vi "rydberg_trigger_snap_2014_8_21_joe.vi"() -> ()   [LabVIEW 2013]
uses:
  AndorCamera/camera_controls.ctl
  <userlib>/atmcd32d.llb/AcquisitionMode_mode typedef.ctl
  <userlib>/atmcd32d.llb/TriggerMode_mode typedef.ctl
  instrumentvi_Neutral/cameratrigger/related_vi/check_pixelfly_status.vi
  <vilib>/Utility/file.llb/Write To Spreadsheet File (I64).vi
panel:
  in  "Num2Save":i32
  in  "Base Filename":string
  in  "Save Files?":bool
  out "appended path 2":path
  out "appended path":path
  in  "Case Constant\n(See Context Help) 2":bool
  in  "Case Constant\n(See Context Help)":bool
  out "iteration#":i32=25
  in  "Turn channels ON/OFF\n(works in real time)":bool[](array[boolean])=[TRUE, TRUE, FALSE, FALSE, FALSE, FALSE, FALSE, FALSE, FALSE, FALSE, FALSE, FALSE, FALSE, FALSE, FALSE, FALSE]
  in  "Save data every nth iteration":dbl=25.0
  out "Analog Input \nVoltage Monitor":T1(graph)={"data[0]"=-0.7588496337314492, "data[1]"=-0.07985869959699164, "data[2]"=0.0, "data[3]"=0.0, "data[4]"=0.0, "data[5]"=0.0, "data[6]"=0.0, "data[7]"=0.0, "data[8]"=0.0, "data[9]"=0.0, "data[10]"=0.0, "data[11]"=0.0, "data[12]"=0.0, "data[13]"=0.0, "data[14]"=0.0, "data[15]"=0.0}
  in  "Tab Control":enum32{"Controls", "Images", "Status"}(tab)=enum."Images"
  in  "Voltage Log File Path":path=path "C:/data/Voltage Log Files/voltagelog011708.txt"
  in  "Monitor voltages?":bool
  in  "Voltage\nMonitor\nControl":u16(ring)=1 caption="Voltage Monitor Control" items=["Off", "Each imaging cycle", "Verdi temp mon"]
  in  "File Path for Atoms":path=path "C:/data/tempfiles/junkatoms.dat"
  in  "File Path for Background":path=path "C:/data/tempfiles/junkback.dat"
  in  "Timeout (min 100 ms)":u32=1000
  in  "Max Iteration (timeout)":i32=51
  in  "Camera background with no image beam.\nIt will be subtracted before the log is taken":i16 min=0
  in  "Software Bin Size":i32=2
  in  "Software Binning?":bool=TRUE
  in  "Cut Image?":bool=TRUE
  in  "ROI Parameters":T2={"Col Start"=250, "Col Stop"=100, "Row Start"=1025, "Row stop"=1000} {"Row stop" min=1 max=1000; "Row Start" min=1 max=1000; "Col Stop" min=1 max=1000; "Col Start" min=1 max=1000}
  in  "Coil Current (amps)":dbl=34.0 format="%.2f"
  in  "Natural Linewidth of Transition (in MHz)":dbl=32.0
  in  "Image Beam Detuning (MHz)":dbl format="%.2f"
  in  "Image Beam Wavelength (m)":dbl=4.61e-07
  in  "Number for Scale":dbl=5.0
  in  "Number of Pixels to Smooth":dbl=1.0
  in  "Cut Borders":dbl
  in  "Limit":dbl=5.0
  in  "Sample Interleave":dbl=1.0 min=1.0
  in  "Pixel Size (m)":dbl=6e-06
  in  "Scale Base Level?":bool
  in  "1D Fit On?":bool=TRUE
  in  "2D Fit On?":bool=TRUE
  in  "Acquisition Parameters":T3={"Acquisition Mode"=enum."Kinetics", "Trigger Mode"=enum."External", "Frame \nTransfer"=FALSE, "Exposure Time (s)"=0.0001, "Accumulation Cycle Time (s)"=0.0, "# Accumulations"=1, "# Kinetics"=2, "Kinetic Cycle Time (s)"=0.0, "Horizontal Bin Size"=1, "Vertical Bin Size"=1} {"Vertical Bin Size" min=1; "Horizontal Bin Size" min=1; "Kinetic Cycle Time (s)" format="%.2f"; "# Kinetics" min=1; "# Accumulations" min=1; "Accumulation Cycle Time (s)" format="%.2f"; "Exposure Time (s)" format="%.2e"}
  out "Andor Initialize Error":errorcluster
  out "?":ext format="%.2f"
  in  "?":i32=35
  in  "?":i32=87
  out "PixelFly Status":bool
  out "Atoms - Background at Analysis Size":dbl[][](graph)
  out "image -  bg sum of ROI from back":dbl(graph)=-492168.0
  out "Last 40 numbers":dbl(graph)
  out "Atoms Image":i32[][](graph)
  out "Atoms - Background":i32[][](graph)
  out "parameters from \npeak absorption":T6={"alpha"=1.0152277070063695e-13, "peakdensity"=4.819850374584978e+17, "alphadenssigzsqrt2pi"=2.914507, "number"=142895.21998245403} {"number" format="%.3e"; "alphadenssigzsqrt2pi" format="%.3e"; "peakdensity" format="%.3e"; "alpha" format="%.3e"}
  out "Image Size for Analysis":i32[](array[numeric])=[150, 100]
  out "peak OD":dbl format="%#_4g"
  in  "# Images to Sum":i32=1
  in  "Continuous Scan?\n(No Images Saved)":bool=TRUE
  in  "Autoscale\nRoutine On?":bool
  in  "Analyze \nImages?":bool=TRUE
  in  "Camera Function":i32(ring)=2 items=["Camera Initialize", "Acquire", "Shutdown"]
  in  "Stop Continuous Scan?":bool
  out "2D Fit Chi-squared":dbl format="%#_3g"
  out "Num Atoms - OD Integral":dbl format="%#_4g"
  out "Num Atoms - Peak OD":dbl format="%#_4g"
  out "Y 1D Fit Values":T7={"Amplitude"=17.90491094333259, "y0"=0.0006453741239587313, "rmswidthy"=3.333942391455422e-05, "offsety"=-3.142553421752575, "Number Y"=176863.40216585185} {"Number Y" format="%.2e"; "offsety" format="%.2e"; "rmswidthy" format="%.2e"; "y0" format="%.2e"; "Amplitude" format="%.2e"}
  out "X 1D Fit Values":T8={"Amplitude"=24.47847782439825, "x0"=0.0009429207504454069, "rmswidthx"=2.376173376668835e-05, "offsetx"=-2.0737454877905925, "Number X"=172333.71575846447} {"Number X" format="%.2e"; "offsetx" format="%.2e"; "rmswidthx" format="%.2e"; "x0" format="%.2e"; "Amplitude" format="%.2e"}
  out "2-D Fit Parameters":T9
  out "Avg Back":ext=1449.7175567626953 format="%.2e"
  out "Avg Atoms-Back":ext=-7.78399887084961 format="%.2e"
  out "Avg Atoms":ext=1441.9335578918458 format="%.2e"
  out "Opticaldepthimagesingle (ln(atoms)-ln(back))(-1)":dbl[][](graph)
  out "Smoothed OD - Fit OD":dbl[][](graph)
  out "Uncut Image - Doubleshot":i32[][](graph)
  out "Y density distribution: log(sum_x atoms) -log(sum_x backgnd)":cluster{dbl[], dbl[]}[](graph)=[{[0.0, 1.2e-05, 2.4e-05, 3.6e-05, 4.8e-05, 6e-05, 7.2e-05, 8.400000000000001e-05, 9.6e-05, 0.000108, 0.00012, 0.000132, 0.000144, 0.000156, 0.00016800000000000002, 0.00018, 0.000192, 0.000204, 0.000216, 0.000228, 0.00024, 0.000252, 0.000264, 0.000276, 0.000288, 0.00030000000000000003, 0.000312, 0.000324, 0.00033600000000000004, 0.000348, 0.00036, 0.000372, 0.000384, 0.00039600000000000003, 0.000408, 0.00042, 0.000432, 0.000444, 0.000456, 0.000468, 0.00048, 0.000492, 0.000504, 0.000516, 0.000528, 0.00054, 0.000552, 0.000564, 0.000576, 0.000588, 0.0006000000000000001, 0.000612, 0.000624, 0.0006360000000000001, 0.000648, 0.00066, 0.0006720000000000001, 0.000684, 0.000696, 0.000708, 0.00072, 0.000732, 0.000744, 0.000756, 0.000768, 0.00078, 0.0007920000000000001, 0.000804, 0.000816, 0.0008280000000000001, 0.00084, 0.000852, 0.000864, 0.000876, 0.000888, 0.0009, 0.000912, 0.000924, 0.000936, 0.0009480000000000001, 0.00096, 0.000972, 0.000984, 0.000996, 0.001008, 0.00102, 0.001032, 0.001044, 0.001056, 0.001068, 0.00108, 0.001092, 0.001104, 0.001116, 0.001128, 0.00114, 0.001152, 0.001164, 0.001176, 0.001188], [-3.3686591448665695, -3.3593416907117444, -2.501141797799619, -3.137266718233832, -3.587719306130566, -2.6390745848241295, -3.6966092446853054, -2.6808187998242374, -3.0319112156403207, -2.7363781603955886, -3.363138854673707, -2.731002614818408, -3.3935197594450983, -3.0493035465378853, -3.2941032756557433, -3.092209549305835, -3.0943983454935733, -3.2393686037710268, -2.730035543135955, -3.287849371356515, -2.5686023814239434, -3.1088703551167782, -2.856653458062283, -3.240447915604136, -3.4894394818825276, -2.9961131164766357, -4.104169957056229, -2.8255474959485127, -3.8878748767015168, -3.0775415698653887, -3.7197529539632797, -3.3776657935209187, -3.8047169273982036, -3.4536401406066943, -3.3930728929356064, -3.1293918380520154, -3.433923718918095, -2.8153587940721536, -3.6029531308467995, -2.4989306176071295, -3.483829652183431, -2.9711985693618317, -3.697510544320039, -3.1132099718149675, -3.803881645787669, -3.6495652439025434, -3.6485837854809233, -3.185441611433589, -1.652208255575033, 0.03140941165247568, 4.4569342541294645, 8.56173788023807, 12.377374823114451, 13.49419715605518, 13.361094012986996, 13.08877719779457, 10.635138116352437, 6.592571400876977, 2.8347368854219894, -0.6335944505865427, -2.5137500326873123, -3.043489857024497, -2.68801842384687, -3.0676047259767074, -2.9163649829733913, -3.168337622954141, -2.7690334242099652, -3.322776293644665, -3.119521162448791, -3.04783132514558, -2.619550840819329, -3.2013707187938962, -2.419650797146687, -2.902692626093767, -3.0917951318126597, -2.8856469922691304, -3.523759843666312, -3.0084041621928463, -3.646833134218241, -3.1529925921761333, -3.371597483779624, -3.5211395371050003, -3.153552371623391, -3.4981555573237983, -3.7751962171532796, -2.992402620435996, -3.2399196976318763, -2.831696410884433, -2.7750651929482046, -2.8873123361618127, -2.360377205045097, -2.399998629312904, -2.590436576132106, -2.2120804438281993, -2.5532249988086733, -2.7154620505466482, -2.369902307173561, -3.201516908291751, -2.571788439326383, -2.629373703639885]}, {[0.0, 1.2e-05, 2.4e-05, 3.6e-05, 4.8e-05, 6e-05, 7.2e-05, 8.400000000000001e-05, 9.6e-05, 0.000108, 0.00012, 0.000132, 0.000144, 0.000156, 0.00016800000000000002, 0.00018, 0.000192, 0.000204, 0.000216, 0.000228, 0.00024, 0.000252, 0.000264, 0.000276, 0.000288, 0.00030000000000000003, 0.000312, 0.000324, 0.00033600000000000004, 0.000348, 0.00036, 0.000372, 0.000384, 0.00039600000000000003, 0.000408, 0.00042, 0.000432, 0.000444, 0.000456, 0.000468, 0.00048, 0.000492, 0.000504, 0.000516, 0.000528, 0.00054, 0.000552, 0.000564, 0.000576, 0.000588, 0.0006000000000000001, 0.000612, 0.000624, 0.0006360000000000001, 0.000648, 0.00066, 0.0006720000000000001, 0.000684, 0.000696, 0.000708, 0.00072, 0.000732, 0.000744, 0.000756, 0.000768, 0.00078, 0.0007920000000000001, 0.000804, 0.000816, 0.0008280000000000001, 0.00084, 0.000852, 0.000864, 0.000876, 0.000888, 0.0009, 0.000912, 0.000924, 0.000936, 0.0009480000000000001, 0.00096, 0.000972, 0.000984, 0.000996, 0.001008, 0.00102, 0.001032, 0.001044, 0.001056, 0.001068, 0.00108, 0.001092, 0.001104, 0.001116, 0.001128, 0.00114, 0.001152, 0.001164, 0.001176, 0.001188], [-3.142553421752575, -3.142553421752575, -3.142553421752575, -3.142553421752575, -3.142553421752575, -3.142553421752575, -3.142553421752575, -3.142553421752575, -3.142553421752575, -3.142553421752575, -3.142553421752575, -3.142553421752575, -3.142553421752575, -3.142553421752575, -3.142553421752575, -3.142553421752575, -3.142553421752575, -3.142553421752575, -3.142553421752575, -3.142553421752575, -3.142553421752575, -3.142553421752575, -3.142553421752575, -3.142553421752575, -3.142553421752575, -3.142553421752575, -3.142553421752575, -3.142553421752575, -3.142553421752575, -3.142553421752575, -3.142553421752573, -3.14255342175253, -3.1425534217517685, -3.1425534217398705, -3.1425534215767574, -3.142553419615115, -3.142553398924452, -3.142553207572838, -3.1425516564361646, -3.1425406396371858, -3.1424721164431455, -3.1420990921048606, -3.1403231424865408, -3.1329354518498045, -3.106116340729864, -3.021287229549591, -2.788007984145684, -2.231927393950265, -1.0878733189191243, 0.9301648516208109, 3.9493125759985808, 7.706020947338827, 11.43621434642004, 14.068401345797076, 14.706907582526853, 13.11971957540532, 9.873322089660576, 6.009141262246697, 2.510273096557114, -0.0751860764137236, -1.680369782741332, -2.530239620690055, -2.917294410160682, -3.0697542735255157, -3.1218850426129303, -3.137398494519852, -3.1414239518658547, -3.1423360201347044, -3.1425166607891493, -3.1425479610692, -3.1425527091570276, -3.142553340061387, -3.1425534135255404, -3.142553421024716, -3.1425534216960047, -3.1425534217487128, -3.142553421752343, -3.142553421752563, -3.1425534217525746, -3.142553421752575, -3.142553421752575, -3.142553421752575, -3.142553421752575, -3.142553421752575, -3.142553421752575, -3.142553421752575, -3.142553421752575, -3.142553421752575, -3.142553421752575, -3.142553421752575, -3.142553421752575, -3.142553421752575, -3.142553421752575, -3.142553421752575, -3.142553421752575, -3.142553421752575, -3.142553421752575, -3.142553421752575, -3.142553421752575, -3.142553421752575]}]
  out "Intensity v/s X":cluster{dbl[], dbl[]}[](graph)=[{[0.0, 1.2e-05, 2.4e-05, 3.6e-05, 4.8e-05, 6e-05, 7.2e-05, 8.400000000000001e-05, 9.6e-05, 0.000108, 0.00012, 0.000132, 0.000144, 0.000156, 0.00016800000000000002, 0.00018, 0.000192, 0.000204, 0.000216, 0.000228, 0.00024, 0.000252, 0.000264, 0.000276, 0.000288, 0.00030000000000000003, 0.000312, 0.000324, 0.00033600000000000004, 0.000348, 0.00036, 0.000372, 0.000384, 0.00039600000000000003, 0.000408, 0.00042, 0.000432, 0.000444, 0.000456, 0.000468, 0.00048, 0.000492, 0.000504, 0.000516, 0.000528, 0.00054, 0.000552, 0.000564, 0.000576, 0.000588, 0.0006000000000000001, 0.000612, 0.000624, 0.0006360000000000001, 0.000648, 0.00066, 0.0006720000000000001, 0.000684, 0.000696, 0.000708, 0.00072, 0.000732, 0.000744, 0.000756, 0.000768, 0.00078, 0.0007920000000000001, 0.000804, 0.000816, 0.0008280000000000001, 0.00084, 0.000852, 0.000864, 0.000876, 0.000888, 0.0009, 0.000912, 0.000924, 0.000936, 0.0009480000000000001, 0.00096, 0.000972, 0.000984, 0.000996, 0.001008, 0.00102, 0.001032, 0.001044, 0.001056, 0.001068, 0.00108, 0.001092, 0.001104, 0.001116, 0.001128, 0.00114, 0.001152, 0.001164, 0.001176, 0.001188, 0.0012000000000000001, 0.001212, 0.001224, 0.0012360000000000001, 0.001248, 0.00126, 0.0012720000000000001, 0.001284, 0.001296, 0.0013080000000000001, 0.00132, 0.001332, 0.0013440000000000001, 0.001356, 0.001368, 0.00138, 0.001392, 0.001404, 0.001416, 0.001428, 0.00144, 0.001452, 0.001464, 0.001476, 0.001488, 0.0015, 0.001512, 0.001524, 0.001536, 0.0015480000000000001, 0.00156, 0.001572, 0.0015840000000000001, 0.001596, 0.001608, 0.0016200000000000001, 0.001632, 0.001644, 0.0016560000000000001, 0.001668, 0.00168, 0.0016920000000000001, 0.001704, 0.001716, 0.001728, 0.00174, 0.001752, 0.001764, 0.001776, 0.001788], [-2.8183440721355737, -2.401522563761773, -2.5237601060707675, -2.500570399573121, -2.506086929574394, -2.3798757992705077, -2.491986345524083, -2.488259685244998, -2.5954764602082605, -2.6088044268195745, -2.565883062250009, -2.640123527845276, -2.5258645679890606, -2.542319425147525, -2.3663141562295777, -2.491158449081013, -2.4827761290987382, -2.5697565230360624, -2.675555471134544, -2.4526500510070264, -2.587401679302161, -2.7170704998887913, -2.5610989943488676, -2.5911334487145723, -2.5002374964478804, -2.4884694389456854, -2.5394904176372393, -2.5500867554972046, -2.378216817131488, -2.5395407567208395, -2.046418844121149, -2.1733857420010736, -2.669858427788313, -2.2304504062857404, -2.586975439308276, -2.4213636413369386, -2.3929041134997533, -2.488418399790703, -2.2930625821045396, -2.6069475160815045, -2.511643300766991, -2.273400532704045, -2.2899489155247466, -2.528198542008795, -2.357612131615724, -2.3432177912642373, -2.3168511287027513, -2.420032372065748, -2.395414080287992, -2.3757390661600084, -2.4716707833126748, -2.2185297028257764, -2.2814791274250865, -2.118623996360043, -2.0182357551965424, -2.432618062946176, -2.230506420081042, -2.146155705062938, -2.3472190640306962, -2.3712543536693147, -2.1875881775472408, -2.1952908358917966, -2.053287952368919, -1.8502300747721847, -1.9848473505809352, -1.9942680470508094, -2.0174521250165753, -2.0969782433525097, -1.8219170436304921, -1.6672326334789886, -1.4869217102946095, -0.9996339197143698, -0.8098748137616667, -0.35967428953222225, -0.650012388682967, 1.7919178156766975, 7.743635801250548, 16.428591835436464, 22.663725551287143, 20.240706904645776, 16.936256193013378, 9.701135845766885, 4.174916332451744, -0.2899352730639748, -1.661331740025389, -1.5080821335172914, -1.9026215949503467, -2.049002401491748, -1.9706402437938095, -2.0311585837459916, -2.077597516112178, -1.930667645093763, -2.1086022731634557, -1.7650030212055299, -1.917311464733416, -1.8111299981898128, -2.075459160990931, -2.2079166808241553, -1.8235763980834463, -1.898222513860219, -1.9621602868612626, -2.0017564868267073, -1.7095965014406147, -2.0323342222595784, -1.6211606697328307, -1.839833902685882, -1.9658503587635323, -1.9776012347161895, -1.887885369120113, -1.9468724100556756, -1.6351243930344026, -1.6613815392586275, -1.6219275265368651, -1.7589024364108354, -1.6045421848466503, -1.8391976965150434, -1.6203149700231734, -1.7969550536250836, -1.5575704192364128, -1.8258635266791998, -1.9097093493073771, -1.8343058761104203, -1.660627277068329, -1.945166122309729, -1.5463727138680952, -1.569489672727741, -1.6225878206881816, -1.7324496472705277, -1.631544148883222, -1.8227215123275755, -1.8797703918872912, -1.8647363562896544, -1.576905869043685, -1.970412155507347, -2.0096411488008243, -1.7813961287674829, -1.8489792019571496, -1.7513334844093151, -1.6826445124467, -1.8905109948545942, -1.7110939804845202, -1.7394070082149256, -1.599355827269278, -1.686777376633131, -1.4884369858077662, -1.653664890583741, -1.8092625318996625, -1.4833808568982931, -1.6619157448002397, -1.371210367738854]}, {[0.0, 1.2e-05, 2.4e-05, 3.6e-05, 4.8e-05, 6e-05, 7.2e-05, 8.400000000000001e-05, 9.6e-05, 0.000108, 0.00012, 0.000132, 0.000144, 0.000156, 0.00016800000000000002, 0.00018, 0.000192, 0.000204, 0.000216, 0.000228, 0.00024, 0.000252, 0.000264, 0.000276, 0.000288, 0.00030000000000000003, 0.000312, 0.000324, 0.00033600000000000004, 0.000348, 0.00036, 0.000372, 0.000384, 0.00039600000000000003, 0.000408, 0.00042, 0.000432, 0.000444, 0.000456, 0.000468, 0.00048, 0.000492, 0.000504, 0.000516, 0.000528, 0.00054, 0.000552, 0.000564, 0.000576, 0.000588, 0.0006000000000000001, 0.000612, 0.000624, 0.0006360000000000001, 0.000648, 0.00066, 0.0006720000000000001, 0.000684, 0.000696, 0.000708, 0.00072, 0.000732, 0.000744, 0.000756, 0.000768, 0.00078, 0.0007920000000000001, 0.000804, 0.000816, 0.0008280000000000001, 0.00084, 0.000852, 0.000864, 0.000876, 0.000888, 0.0009, 0.000912, 0.000924, 0.000936, 0.0009480000000000001, 0.00096, 0.000972, 0.000984, 0.000996, 0.001008, 0.00102, 0.001032, 0.001044, 0.001056, 0.001068, 0.00108, 0.001092, 0.001104, 0.001116, 0.001128, 0.00114, 0.001152, 0.001164, 0.001176, 0.001188, 0.0012000000000000001, 0.001212, 0.001224, 0.0012360000000000001, 0.001248, 0.00126, 0.0012720000000000001, 0.001284, 0.001296, 0.0013080000000000001, 0.00132, 0.001332, 0.0013440000000000001, 0.001356, 0.001368, 0.00138, 0.001392, 0.001404, 0.001416, 0.001428, 0.00144, 0.001452, 0.001464, 0.001476, 0.001488, 0.0015, 0.001512, 0.001524, 0.001536, 0.0015480000000000001, 0.00156, 0.001572, 0.0015840000000000001, 0.001596, 0.001608, 0.0016200000000000001, 0.001632, 0.001644, 0.0016560000000000001, 0.001668, 0.00168, 0.0016920000000000001, 0.001704, 0.001716, 0.001728, 0.00174, 0.001752, 0.001764, 0.001776, 0.001788], [-2.0737454877905925, -2.0737454877905925, -2.0737454877905925, -2.0737454877905925, -2.0737454877905925, -2.0737454877905925, -2.0737454877905925, -2.0737454877905925, -2.0737454877905925, -2.0737454877905925, -2.0737454877905925, -2.0737454877905925, -2.0737454877905925, -2.0737454877905925, -2.0737454877905925, -2.0737454877905925, -2.0737454877905925, -2.0737454877905925, -2.0737454877905925, -2.0737454877905925, -2.0737454877905925, -2.0737454877905925, -2.0737454877905925, -2.0737454877905925, -2.0737454877905925, -2.0737454877905925, -2.0737454877905925, -2.0737454877905925, -2.0737454877905925, -2.0737454877905925, -2.0737454877905925, -2.0737454877905925, -2.0737454877905925, -2.0737454877905925, -2.0737454877905925, -2.0737454877905925, -2.0737454877905925, -2.0737454877905925, -2.0737454877905925, -2.0737454877905925, -2.0737454877905925, -2.0737454877905925, -2.0737454877905925, -2.0737454877905925, -2.0737454877905925, -2.0737454877905925, -2.0737454877905925, -2.0737454877905925, -2.0737454877905925, -2.0737454877905925, -2.0737454877905925, -2.0737454877905925, -2.0737454877905925, -2.0737454877905925, -2.0737454877905925, -2.0737454877905925, -2.0737454877905925, -2.0737454877905925, -2.0737454877905925, -2.0737454877905925, -2.0737454877905925, -2.0737454877905925, -2.073745487790578, -2.073745487789698, -2.073745487748773, -2.0737454862751323, -2.073745445235809, -2.0737445618346193, -2.073729875366191, -2.073541507399717, -2.0716803713160936, -2.0575446026371003, -1.9752602822028478, -1.6098273966897678, -0.3803839855887031, 2.715820000636734, 8.423627049166667, 15.754276644617699, 21.388186935825832, 21.85183342897553, 16.8322343699678, 9.50266684232387, 3.41896670995723, -0.05427383695049559, -1.4984026137046382, -1.9467308492977926, -2.052017531704562, -2.0708652918518737, -2.0734496434587752, -2.0737219404138356, -2.0737440354787706, -2.073745418381675, -2.073745485220145, -2.0737454877168293, -2.073745487788952, -2.073745487790564, -2.073745487790592, -2.0737454877905925, -2.0737454877905925, -2.0737454877905925, -2.0737454877905925, -2.0737454877905925, -2.0737454877905925, -2.0737454877905925, -2.0737454877905925, -2.0737454877905925, -2.0737454877905925, -2.0737454877905925, -2.0737454877905925, -2.0737454877905925, -2.0737454877905925, -2.0737454877905925, -2.0737454877905925, -2.0737454877905925, -2.0737454877905925, -2.0737454877905925, -2.0737454877905925, -2.0737454877905925, -2.0737454877905925, -2.0737454877905925, -2.0737454877905925, -2.0737454877905925, -2.0737454877905925, -2.0737454877905925, -2.0737454877905925, -2.0737454877905925, -2.0737454877905925, -2.0737454877905925, -2.0737454877905925, -2.0737454877905925, -2.0737454877905925, -2.0737454877905925, -2.0737454877905925, -2.0737454877905925, -2.0737454877905925, -2.0737454877905925, -2.0737454877905925, -2.0737454877905925, -2.0737454877905925, -2.0737454877905925, -2.0737454877905925, -2.0737454877905925, -2.0737454877905925, -2.0737454877905925, -2.0737454877905925, -2.0737454877905925, -2.0737454877905925, -2.0737454877905925, -2.0737454877905925, -2.0737454877905925]}] caption="X Density Distribution: log(sum_y atoms) -log(sum_y backgnd)"
  out "Background Image":i32[][](graph)
  out "Strip Chart\nerror out":errorcluster
  in  "Strip Chart\nerror in":errorcluster
  out "Strip chart counter":dbl
  out "error out":errorcluster={"status"=TRUE, "code"=-131, "source"="Remove buffer from list.vi: Picture buffer already in use"} caption="Camera Error Out 1"
  out "V bin 2":i32(ring) items=["1", "2"]
  out "H bin 2":i32(ring) items=["1", "2"]
  out "Size":i32=5242880
  out "Camera Information":T10 {"VS Speed (us)" format="%.2f"}
  out "Output ClusterY\n(arb fit)":T11={"amplitudey"=0.008995711509471623, "temperaturey"=0.002709094402736608, "alphay"=0.0011778671316246122, "offsety"=-0.0002344292151486787, "numbery"=771798750.645837, "peakdensityy"=4696134676573208.0, "centery"=0.004923587672892697} {"centery" format="%.2e"; "peakdensityy" format="%.2e"; "numbery" format="%.2e"; "offsety" format="%.2e"; "alphay" format="%.2e"; "temperaturey" format="%.2e"; "amplitudey" format="%.2e"}
  out "Output Cluster X\n(arb fit)":T12={"amplitudex"=0.0047697219685124154, "temperaturex"=0.0023439442598952344, "alphax"=0.0010191061999544498, "offsetx"=8.440276213188199e-05, "numberx"=708132868.1536969, "peakdensityx"=6652452808873044.0, "centerx"=0.0037182148271134325} {"centerx" format="%.2e"; "peakdensityx" format="%.2e"; "numberx" format="%.2e"; "offsetx" format="%.2e"; "alphax" format="%.2e"; "temperaturex" format="%.2e"; "amplitudex" format="%.2e"}
  out "Y side(by arbfit)":cluster{cluster{dbl, dbl}[]}[](graph)=[{[{0.0, -9.666143798828125e-05}, {4.63e-05, 4.321251220703125e-05}, {9.26e-05, -0.00016961046142578126}, {0.00013890000000000002, -0.0001606823974609375}, {0.0001852, -3.920782470703125e-05}, {0.0002315, -0.000111915087890625}, {0.00027780000000000003, -0.00018772257080078126}, {0.0003241, -0.00014607723388671877}, {0.0003704, 3.730218505859375e-05}, {0.0004167, -0.000120493310546875}, {0.000463, -2.0831201171875e-05}, {0.0005093, 8.1265576171875e-05}, {0.0005556000000000001, -4.6981127929687503e-05}, {0.0006019, 2.730753173828125e-05}, {0.0006482, 0.0001042299560546875}, {0.0006945, 8.897061767578125e-05}, {0.0007408, -0.0001128991943359375}, {0.0007871, -3.39658935546875e-05}, {0.0008334, 0.00021708648681640627}, {0.0008797, 1.521951904296875e-05}, {0.000926, -8.81429443359375e-05}, {0.0009723, 0.00017849017333984376}, {0.0010186, 0.00016118013916015624}, {0.0010649, 4.3130029296875e-05}, {0.0011112000000000001, 0.000101584814453125}, {0.0011575000000000001, 0.0001667121826171875}, {0.0012038, 0.0001330364013671875}, {0.0012501, 1.435771484375e-05}, {0.0012964, 0.00013017509765625}, {0.0013427, 0.0001979874267578125}, {0.001389, 0.0001995517578125}, {0.0014353, 5.386134033203125e-05}, {0.0014816, 0.00013825557861328125}, {0.0015279, 0.00037487060546875003}, {0.0015742, 0.0001915253173828125}, {0.0016205, 0.000173282373046875}, {0.0016668, 0.00030387272949218753}, {0.0017131, 0.0005522344604492188}, {0.0017594, 0.0003743757080078125}, {0.0018057, 0.000244183544921875}, {0.001852, 0.0004390764404296875}, {0.0018983000000000001, 0.0004536360961914063}, {0.0019446, 0.00044938680419921874}, {0.0019909, 0.00031516435546875}, {0.0020372, 0.0003973002685546875}, {0.0020835, 0.000558414990234375}, {0.0021298, 0.0005315966674804687}, {0.0021761, 0.00047105989990234374}, {0.0022224000000000002, 0.0006024039794921875}, {0.0022687000000000002, 0.0006190456176757812}, {0.0023150000000000002, 0.0006605089233398438}, {0.0023613, 0.0006151063476562501}, {0.0024076, 0.0007049785888671875}, {0.0024539, 0.0008554387939453125}, {0.0025002, 0.000755099755859375}, {0.0025465, 0.0008008635498046875}, {0.0025928, 0.0007846542358398437}, {0.0026391, 0.00092633427734375}, {0.0026854, 0.0009349409423828125}, {0.0027317, 0.0009390679321289063}, {0.002778, 0.0009715178466796875}, {0.0028243, 0.0009944736938476563}, {0.0028706, 0.001180484033203125}, {0.0029169, 0.0010933195068359375}, {0.0029632, 0.0010906231689453126}, {0.0030095, 0.0010906317016601563}, {0.0030558, 0.0013240981567382813}, {0.0031021, 0.0014536930297851564}, {0.0031484, 0.001447785546875}, {0.0031947, 0.0013987793212890626}, {0.003241, 0.0015179443725585938}, {0.0032873, 0.0015591374755859375}, {0.0033336, 0.0016731800537109376}, {0.0033799, 0.0016079417602539064}, {0.0034262, 0.0015991075561523438}, {0.0034725, 0.0018513971801757813}, {0.0035188, 0.0018405805419921875}, {0.0035651, 0.0018605926025390626}, {0.0036114, 0.001904240283203125}, {0.0036577, 0.0018782012817382813}, {0.003704, 0.0019519751342773437}, {0.0037503000000000002, 0.0020929782470703127}, {0.0037966000000000002, 0.002198195153808594}, {0.0038429000000000002, 0.0021514216552734377}, {0.0038892, 0.0020961069091796876}, {0.0039355, 0.002265489831542969}, {0.0039818, 0.0023468663330078127}, {0.0040281, 0.002427193310546875}, {0.0040744, 0.0024689637939453125}, {0.0041207, 0.0024438804565429686}, {0.004167, 0.0024601580322265626}, {0.0042133, 0.002636688525390625}, {0.0042596, 0.002699147998046875}, {0.0043059, 0.002643045397949219}, {0.0043522, 0.0026505143676757814}, {0.0043985, 0.0026222966796875}, {0.0044448000000000005, 0.0027097114990234377}, {0.0044911000000000005, 0.0027219531005859376}, {0.0045374000000000005, 0.0027993960205078125}, {0.0045837000000000004, 0.002850597998046875}, {0.0046300000000000004, 0.0028023995361328127}, {0.0046763, 0.0027945295288085937}, {0.0047226, 0.0029437581787109374}, {0.0047689, 0.0029110010864257813}, {0.0048152, 0.0030008591064453125}, {0.0048615, 0.002974151708984375}, {0.0049078, 0.002937995751953125}, {0.0049541, 0.0029096813598632814}, {0.0050004, 0.0029673767333984378}, {0.0050467, 0.003066478527832031}, {0.005093, 0.00306333564453125}, {0.0051393, 0.003041998168945313}, {0.0051856, 0.0028867596435546874}, {0.0052319, 0.0027757006713867187}, {0.0052782, 0.0028882158935546877}, {0.0053245, 0.0029104151733398437}, {0.0053708, 0.0027892534667968752}, {0.0054171, 0.0027464476806640624}, {0.0054634, 0.002764500061035156}, {0.0055097, 0.0026023215942382813}, {0.005556, 0.0025186128173828124}, {0.0056023, 0.002569339807128906}, {0.0056486, 0.0024484426147460938}, {0.0056949, 0.0024748428344726564}, {0.0057412, 0.002454739758300781}, {0.0057875, 0.0023008465576171877}, {0.0058338, 0.0023179062988281252}, {0.0058801, 0.00228233056640625}, {0.0059264, 0.0022157355712890624}, {0.0059727, 0.0020830091918945313}, {0.006019, 0.002083563818359375}, {0.0060653, 0.0020847953735351563}, {0.0061116, 0.002062195056152344}, {0.0061579, 0.0019736823608398437}, {0.0062042, 0.0018520598876953125}, {0.0062505, 0.0018948542968750001}, {0.0062968, 0.0017422921997070314}, {0.0063431, 0.0016028676391601562}, {0.0063894, 0.0016803645996093751}, {0.0064357, 0.0015904127197265625}, {0.006482, 0.0015004665283203126}, {0.0065283, 0.001450151953125}, {0.0065746, 0.0014172981567382812}, {0.0066209, 0.001336484814453125}, {0.0066672, 0.00135934111328125}, {0.0067135, 0.001208789892578125}, {0.0067598, 0.0012902744750976562}, {0.0068061, 0.0011487451782226563}, {0.0068524, 0.001103211767578125}, {0.0068987, 0.0011628611328125}, {0.006945, 0.0011180217163085937}, {0.0069913, 0.00104233369140625}, {0.0070376, 0.001006120849609375}, {0.0070839, 0.0009368323608398438}, {0.0071302, 0.0008879626586914063}, {0.0071765, 0.0008855393676757813}, {0.0072228, 0.0007939548950195313}, {0.0072691, 0.0007488623413085938}, {0.0073154, 0.0007369250732421875}, {0.0073617, 0.0007228916015625}, {0.007408, 0.0006716412719726563}, {0.0074543000000000005, 0.0006353601684570313}, {0.0075006000000000005, 0.0006309515991210938}, {0.0075469000000000005, 0.0005209734375}, {0.0075932000000000005, 0.0005503174438476563}, {0.0076395000000000005, 0.0005640096069335937}, {0.0076858000000000004, 0.0005803668212890625}, {0.0077321, 0.00046943583984375}, {0.0077784, 0.0004919138549804688}, {0.0078247, 0.0004567334716796875}, {0.007871, 0.0004032162841796875}, {0.0079173, 0.0003256823486328125}, {0.0079636, 0.00034895675048828126}, {0.0080099, 0.0002296722412109375}, {0.0080562, 0.00032278122558593753}, {0.0081025, 0.00024264196777343752}, {0.0081488, 0.0002704131103515625}, {0.0081951, 0.0002514306640625}, {0.0082414, 0.00023038614501953125}, {0.0082877, 0.00023180257568359376}]}, {[{0.0, -0.00010865906187833456}, {4.63e-05, -0.00010248175881259633}, {9.26e-05, -9.60946713894237e-05}, {0.00013890000000000002, -8.949093944564066e-05}, {0.0001852, -8.266349606890666e-05}, {0.0002315, -7.560506264006202e-05}, {0.00027780000000000003, -6.830814386093194e-05}, {0.0003241, -6.076502277862111e-05}, {0.0003704, -5.296775581859711e-05}, {0.0004167, -4.4908167840241404e-05}, {0.000463, -3.657784723005229e-05}, {0.0005093, -2.7968141049325046e-05}, {0.0005556000000000001, -1.9070150254923014e-05}, {0.0006019, -9.874725013701312e-06}, {0.0006482, -3.724601332668094e-07}, {0.0006945, 9.446309365930862e-06}, {0.0007408, 1.9591512509667256e-05}, {0.0007871, 3.0073346429921213e-05}, {0.0008334, 4.090228019253389e-05}, {0.0008797, 5.2089058356076504e-05}, {0.000926, 6.364470422192584e-05}, {0.0009723, 7.558052273170855e-05}, {0.0010186, 8.79081029641e-05}, {0.0010649, 0.00010063932017842472}, {0.0011112000000000001, 0.00011378633734756733}, {0.0011575000000000001, 0.0001273616061173385}, {0.0012038, 0.00014137786712360722}, {0.0012501, 0.00015584814959217083}, {0.0012964, 0.00017078577013944924}, {0.0013427, 0.0001862043306846068}, {0.001389, 0.00020211771537558232}, {0.0014353, 0.00021854008642268471}, {0.0014816, 0.00023548587872383942}, {0.0015279, 0.00025296979315517985}, {0.0015742, 0.00027100678838941274}, {0.0016205, 0.00028961207109216836}, {0.0016668, 0.00030880108433330974}, {0.0017131, 0.00032858949403583845}, {0.0017594, 0.0003489931732695157}, {0.0018057, 0.00037002818417953464}, {0.001852, 0.0003917107573224413}, {0.0018983000000000001, 0.00041405726816191505}, {0.0019446, 0.00043708421045589795}, {0.0019909, 0.00046080816624380496}, {0.0020372, 0.00048524577211806353}, {0.0020835, 0.0005104136814379354}, {0.0021298, 0.0005363285221153792}, {0.0021761, 0.0005630068495725409}, {0.0022224000000000002, 0.0005904650944382619}, {0.0022687000000000002, 0.0006187195045167119}, {0.0023150000000000002, 0.0006477860805248956}, {0.0023613, 0.0006776805050573274}, {0.0024076, 0.0007084180641957342}, {0.0024539, 0.000740013561139293}, {0.0025002, 0.0007724812211868801}, {0.0025465, 0.0008058345873573525}, {0.0025928, 0.0008400864058874109}, {0.0026391, 0.0008752485007996484}, {0.0026854, 0.0009113316366866587}, {0.0027317, 0.0009483453688115168}, {0.002778, 0.0009862978795816956}, {0.0028243, 0.0010251958004140647}, {0.0028706, 0.0010650440179748686}, {0.0029169, 0.0011058454637528246}, {0.0029632, 0.0011476008859085435}, {0.0030095, 0.0011903086023428125}, {0.0030558, 0.0012339642339440908}, {0.0031021, 0.0012785604170168652}, {0.0031484, 0.0013240864939633146}, {0.0031947, 0.0013705281813981287}, {0.003241, 0.0014178672150286608}, {0.0032873, 0.001466080970839556}, {0.0033336, 0.0015151420623937199}, {0.0033799, 0.0015650179144126902}, {0.0034262, 0.0016156703132432844}, {0.0034725, 0.001667054935369524}, {0.0035188, 0.0017191208558060519}, {0.0035651, 0.0017718100390292427}, {0.0036114, 0.0018250568160826273}, {0.0036577, 0.0018787873526509141}, {0.003704, 0.0019329191142461635}, {0.0037503000000000002, 0.00198736033620042}, {0.0037966000000000002, 0.0020420095079141044}, {0.0038429000000000002, 0.0020967548827606724}, {0.0038892, 0.0021514740271722454}, {0.0039355, 0.0022060334246843507}, {0.0039818, 0.0022602881530293956}, {0.0040281, 0.0023140816546324302}, {0.0040744, 0.002367245622930107}, {0.0041207, 0.0024196000286033858}, {0.004167, 0.002470953310823123}, {0.0042133, 0.002521102758619363}, {0.0042596, 0.0025698351060790066}, {0.0043059, 0.0026169273617292817}, {0.0043522, 0.002662147886520171}, {0.0043985, 0.0027052577254283307}, {0.0044448000000000005, 0.0027460121836947304}, {0.0044911000000000005, 0.002784162618292176}, {0.0045374000000000005, 0.0028194583853482155}, {0.0045837000000000004, 0.0028516488390996934}, {0.0046300000000000004, 0.002880485205228244}, {0.0046763, 0.0029057220225760993}, {0.0047226, 0.0029271175887845657}, {0.0047689, 0.0029444322413275594}, {0.0048152, 0.002957421587936099}, {0.0048615, 0.0029658152533030583}, {0.0049078, 0.002969223498278089}, {0.0049541, 0.0029668701892216977}, {0.0050004, 0.0029593929253844222}, {0.0050467, 0.00294726075821299}, {0.005093, 0.002930754675653734}, {0.0051393, 0.0029101216222434004}, {0.0051856, 0.0028856014002929618}, {0.0052319, 0.0028574350907477806}, {0.0052782, 0.002825867425137388}, {0.0053245, 0.0027911466346986157}, {0.0053708, 0.002753523144018291}, {0.0054171, 0.002713247751183462}, {0.0054634, 0.002670569636241478}, {0.0055097, 0.0026257343940900416}, {0.005556, 0.002578982207448093}, {0.0056023, 0.0025305462263872317}, {0.0056486, 0.002480651188686202}, {0.0056949, 0.002429512293337682}, {0.0057412, 0.002377334324465013}, {0.0057875, 0.0023243110127359433}, {0.0058338, 0.002270624614829798}, {0.0058801, 0.0022164456877257805}, {0.0059264, 0.0021619330328464833}, {0.0059727, 0.002107233784866407}, {0.006019, 0.0020524836208415213}, {0.0060653, 0.001997807066881443}, {0.0061116, 0.0019433178815944}, {0.0061579, 0.0018891194977744344}, {0.0062042, 0.0018353055061120958}, {0.0062505, 0.001781960166980848}, {0.0062968, 0.0017291589385044904}, {0.0063431, 0.0016769690110975607}, {0.0063894, 0.0016254498404642377}, {0.0064357, 0.0015746536726311895}, {0.006482, 0.0015246260559770423}, {0.0065283, 0.0014754063364144769}, {0.0065746, 0.0014270281328940674}, {0.0066209, 0.0013795197912482894}, {0.0066672, 0.0013329048150973063}, {0.0067135, 0.0012872022731128603}, {0.0067598, 0.0012424271823999015}, {0.0068061, 0.0011985908681233519}, {0.0068524, 0.0011557012997941273}, {0.0068987, 0.0011137634048471732}, {0.006945, 0.0010727793603062688}, {0.0069913, 0.0010327488634456659}, {0.0070376, 0.0009936693824358488}, {0.0070839, 0.0009555363880071484}, {0.0071302, 0.000918343567186836}, {0.0071765, 0.0008820830201678386}, {0.0072228, 0.000846745441354734}, {0.0072691, 0.0008123202856087498}, {0.0073154, 0.0007787959206810894}, {0.0073617, 0.0007461597667854064}, {0.007408, 0.0007143984242176186}, {0.0074543000000000005, 0.0006834977898860251}, {0.0075006000000000005, 0.0006534431635681152}, {0.0075469000000000005, 0.0006242193446634763}, {0.0075932000000000005, 0.0005958107201656227}, {0.0076395000000000005, 0.0005682013445298609}, {0.0076858000000000004, 0.0005413750120699895}, {0.0077321, 0.0005153153224739417}, {0.0077784, 0.0004900057399876574}, {0.0078247, 0.00046542964677764}, {0.007871, 0.00044157039094588804}, {0.0079173, 0.0004184113296362065}, {0.0079636, 0.00039593586763832716}, {0.0080099, 0.00037412749186567767}, {0.0080562, 0.0003529698020541209}, {0.0081025, 0.0003324465380022771}, {0.0081488, 0.00031254160364927336}, {0.0081951, 0.0002932390882626329}, {0.0082414, 0.0002745232849876373}, {0.0082877, 0.00025637870698957466}]}]
  out "X  side(by arbfit)":cluster{cluster{dbl, dbl}[]}[](graph)=[{[{0.0, 0.000743761572265625}, {2.33e-05, 0.0007473872375488281}, {4.66e-05, 0.0007493540832519531}, {6.99e-05, 0.0007557293762207032}, {9.32e-05, 0.0007686240844726563}, {0.0001165, 0.00077954912109375}, {0.0001398, 0.0007826209045410156}, {0.0001631, 0.0007907256652832031}, {0.0001864, 0.0007821574523925782}, {0.0002097, 0.0007862804809570312}, {0.000233, 0.0008101708740234375}, {0.0002563, 0.0008241846496582032}, {0.0002796, 0.0008290000305175781}, {0.0003029, 0.0008148449584960938}, {0.0003262, 0.0008321311584472657}, {0.0003495, 0.0008452745483398437}, {0.0003728, 0.0008275051147460938}, {0.00039610000000000003, 0.0008584829345703126}, {0.0004194, 0.0008749270080566406}, {0.0004427, 0.000853769287109375}, {0.000466, 0.0008967488220214844}, {0.0004893, 0.0008642676086425781}, {0.0005126, 0.0008836195617675782}, {0.0005359, 0.0009061874206542969}, {0.0005592, 0.0008940415832519532}, {0.0005825, 0.00090533681640625}, {0.0006058, 0.0009135320068359375}, {0.0006291000000000001, 0.0009309453735351562}, {0.0006524, 0.0009473527099609375}, {0.0006757, 0.0009284755126953125}, {0.000699, 0.0009535895324707032}, {0.0007223, 0.0009482033142089844}, {0.0007456, 0.0009242337951660156}, {0.0007689, 0.0009652351806640625}, {0.0007922000000000001, 0.0009666396667480469}, {0.0008155, 0.0009782401000976563}, {0.0008388, 0.0009873198059082032}, {0.0008621, 0.0009737129638671875}, {0.0008854, 0.0010071917297363282}, {0.0009087, 0.0009977870422363281}, {0.000932, 0.000999587158203125}, {0.0009553000000000001, 0.0010326335571289062}, {0.0009786, 0.0010125129516601562}, {0.0010019, 0.0010295589477539063}, {0.0010252, 0.0010326561645507813}, {0.0010485, 0.0010313138488769532}, {0.0010718, 0.00106711552734375}, {0.0010951000000000001, 0.0010514740173339844}, {0.0011184, 0.001073459735107422}, {0.0011417, 0.0010450874206542969}, {0.001165, 0.0010686669616699219}, {0.0011883, 0.0010922125915527345}, {0.0012116, 0.0010816097106933593}, {0.0012349, 0.00110401083984375}, {0.0012582000000000001, 0.0011046042846679688}, {0.0012815, 0.0010739768798828126}, {0.0013048, 0.001109360321044922}, {0.0013281, 0.0011030161132812501}, {0.0013514, 0.0011219272216796876}, {0.0013747, 0.0011355453674316406}, {0.001398, 0.0011239336303710938}, {0.0014213000000000001, 0.0011469960266113281}, {0.0014446, 0.00115329501953125}, {0.0014679, 0.0011437377319335937}, {0.0014912, 0.0011699453857421875}, {0.0015145, 0.0011587010192871093}, {0.0015378, 0.0011873615783691406}, {0.0015611, 0.0011859260070800782}, {0.0015844000000000001, 0.0011899388244628907}, {0.0016077, 0.0012199812622070312}, {0.001631, 0.0011976168701171876}, {0.0016543, 0.0012130266540527344}, {0.0016776, 0.0012230784790039063}, {0.0017009, 0.0012087453735351564}, {0.0017242, 0.001240130126953125}, {0.0017475000000000001, 0.0012251385803222657}, {0.0017708, 0.001247861865234375}, {0.0017941, 0.0012577752197265625}, {0.0018174, 0.00125819345703125}, {0.0018407, 0.001266142791748047}, {0.001864, 0.001258614520263672}, {0.0018873, 0.001270243212890625}, {0.0019106000000000001, 0.0012918728637695313}, {0.0019339000000000001, 0.0012865685974121095}, {0.0019572, 0.0013176029357910156}, {0.0019805, 0.0012929099792480469}, {0.0020038, 0.0012978412231445312}, {0.0020271, 0.0013366722961425782}, {0.0020504, 0.0013322327636718751}, {0.0020737, 0.0013488068298339844}, {0.002097, 0.0013553488525390625}, {0.0021203, 0.0013148787414550781}, {0.0021436, 0.001352384454345703}, {0.0021669000000000002, 0.001340054931640625}, {0.0021902000000000002, 0.0013639933654785157}, {0.0022135, 0.001393996240234375}, {0.0022368, 0.0013536843811035157}, {0.0022601, 0.0014101944580078125}, {0.0022834, 0.0013983396911621095}, {0.0023067, 0.0013908735900878906}, {0.00233, 0.001449927001953125}, {0.0023533, 0.0014175955627441406}, {0.0023766, 0.0014422602600097656}, {0.0023999, 0.0014375042236328126}, {0.0024232, 0.00143208974609375}, {0.0024465, 0.0014523120849609375}, {0.0024698, 0.001446640447998047}, {0.0024931000000000003, 0.0014835838012695313}, {0.0025164000000000002, 0.001486641455078125}, {0.0025397, 0.001466512371826172}, {0.002563, 0.0015129310607910156}, {0.0025863, 0.0014776069641113281}, {0.0026096, 0.001518209893798828}, {0.0026329, 0.0015192978759765625}, {0.0026562, 0.001507657879638672}, {0.0026795, 0.0015395258666992188}, {0.0027028, 0.001535609130859375}, {0.0027261, 0.0015412016418457032}, {0.0027494, 0.0015846870178222656}, {0.0027727, 0.001561531365966797}, {0.002796, 0.0015878379272460939}, {0.0028193000000000003, 0.0015632919189453125}, {0.0028426000000000002, 0.0015500665771484374}, {0.0028659000000000002, 0.0015918055297851562}, {0.0028892, 0.0015806628967285157}, {0.0029125, 0.0016097416931152343}, {0.0029358, 0.0016191096435546875}, {0.0029591, 0.0015954538024902344}, {0.0029824, 0.0016432628479003907}, {0.0030057, 0.0016260953369140625}, {0.003029, 0.00164577509765625}, {0.0030523, 0.0016838714294433593}, {0.0030756, 0.0016387018005371095}, {0.0030989, 0.0016684023010253906}, {0.0031222, 0.0016431102478027344}, {0.0031455, 0.0016455829345703124}, {0.0031688000000000003, 0.001683786651611328}, {0.0031921000000000002, 0.0016447379821777344}, {0.0032154, 0.0016845326965332032}, {0.0032387, 0.001670273065185547}, {0.003262, 0.0016631234680175781}, {0.0032853, 0.0016912329711914064}, {0.0033086, 0.0016726383666992187}, {0.0033319, 0.0017014034851074219}, {0.0033552, 0.0017117181213378906}, {0.0033785, 0.001680921160888672}, {0.0034018, 0.001689528936767578}, {0.0034251, 0.0016496296630859376}, {0.0034484, 0.0016748143310546875}, {0.0034717, 0.00170410224609375}, {0.0034950000000000003, 0.0016960681335449219}, {0.0035183000000000002, 0.0017076120483398437}, {0.0035416, 0.0016810313720703124}, {0.0035649, 0.0016637649536132813}, {0.0035882, 0.0017159457092285157}, {0.0036115, 0.0017127778442382812}, {0.0036348, 0.0017286002136230468}, {0.0036581, 0.0017005924438476562}, {0.0036814, 0.0016708269470214845}, {0.0037047, 0.0017170449951171875}, {0.003728, 0.0017033675048828125}, {0.0037513, 0.0017282554504394533}, {0.0037746, 0.0017212443237304687}, {0.0037979, 0.0016697333129882812}, {0.0038212000000000003, 0.001710907080078125}, {0.0038445000000000003, 0.0017063064697265624}, {0.0038678000000000002, 0.0017241889404296874}, {0.0038911, 0.0017277524353027343}, {0.0039144, 0.0016877853393554687}, {0.0039377, 0.0017066512329101562}, {0.003961, 0.0016772078918457032}, {0.0039843000000000005, 0.0016903230224609375}, {0.0040076, 0.001713213037109375}, {0.0040309000000000005, 0.0016570618530273437}, {0.0040542, 0.0017010530700683594}, {0.0040775, 0.0016834475402832032}, {0.0041008, 0.0016736924377441407}, {0.0041241, 0.0016988092834472656}, {0.0041474, 0.0016336999084472657}, {0.0041707, 0.001666085040283203}, {0.004194, 0.0016937621765136719}, {0.0042173, 0.001654040936279297}, {0.0042406, 0.0016648981506347657}, {0.0042639, 0.0016372492736816406}, {0.0042872, 0.0016537752990722656}, {0.0043105, 0.0016855132934570313}, {0.0043338000000000005, 0.0016447662414550781}, {0.0043571, 0.0016486038513183593}, {0.0043804000000000004, 0.0016160406860351562}, {0.0044037, 0.001606876202392578}, {0.004427, 0.0016453314270019532}, {0.0044503, 0.0015990257751464843}, {0.0044736, 0.0016388770080566406}, {0.0044969, 0.0016056949645996093}, {0.0045202, 0.0015764776977539063}, {0.0045435, 0.0016024140625}, {0.0045668, 0.00157939970703125}, {0.0045901, 0.0015959342102050782}, {0.0046134, 0.0015723857543945314}, {0.0046367, 0.0015299487976074219}, {0.00466, 0.0015728011657714844}, {0.0046833000000000005, 0.0015347557006835937}, {0.0047066, 0.0015534746459960939}, {0.0047299, 0.0015743017333984374}, {0.0047532, 0.00152224814453125}, {0.0047765, 0.0015386130920410157}, {0.0047998, 0.00151447119140625}, {0.0048231, 0.0015109105224609374}, {0.0048464, 0.001534764178466797}, {0.0048697, 0.0014920078918457032}, {0.004893, 0.001510981170654297}, {0.0049163, 0.001462451513671875}, {0.0049396, 0.001448163623046875}, {0.0049629, 0.0014723676940917969}, {0.0049862000000000005, 0.0014467167480468751}, {0.0050095, 0.00146563916015625}, {0.0050328000000000005, 0.0014707766967773437}, {0.0050561, 0.0014142864013671876}, {0.0050794, 0.0014555364685058594}, {0.0051027, 0.0014017421081542968}, {0.005126, 0.001429526629638672}, {0.0051493, 0.0014398412658691406}, {0.0051726, 0.0014118815368652344}, {0.0051959, 0.0014256777160644532}, {0.0052192, 0.0013943607849121094}, {0.0052425, 0.0013844615600585937}, {0.0052658, 0.0014051558288574219}, {0.0052891, 0.0013652085144042969}, {0.0053124, 0.0013914924682617187}, {0.0053357000000000005, 0.0013450879089355469}, {0.005359, 0.001346430224609375}, {0.0053823000000000005, 0.0013769841552734375}, {0.0054056, 0.0013242636474609375}, {0.0054289, 0.0013574202575683595}, {0.0054522, 0.0013375342041015625}, {0.0054755, 0.001303204833984375}, {0.0054988, 0.001341041180419922}, {0.0055221, 0.0013077743591308594}, {0.0055454, 0.0013125134399414062}, {0.0055687, 0.0013193634887695312}, {0.005592, 0.0012819566833496094}, {0.0056153, 0.0012987172607421876}, {0.0056386000000000006, 0.0012782999328613282}, {0.0056619, 0.0012642098571777345}, {0.0056852000000000005, 0.0012895386474609375}, {0.0057085, 0.0012464008605957031}, {0.0057318000000000004, 0.0012559864074707032}, {0.0057551, 0.0012403646789550782}, {0.0057784, 0.0012355719055175782}, {0.0058017, 0.00124119267578125}, {0.005825, 0.0012141711547851563}, {0.0058483, 0.0012365383728027343}, {0.0058716, 0.0012224624267578126}, {0.0058949, 0.0011948050720214844}, {0.0059182, 0.0012144452697753906}, {0.0059415, 0.0012016692504882812}, {0.0059648, 0.001197537744140625}, {0.0059881000000000005, 0.0011997447937011718}, {0.0060114, 0.001165172393798828}, {0.0060347000000000005, 0.0011889497497558593}, {0.006058, 0.0011639459411621094}, {0.0060813, 0.001137167449951172}, {0.0061046, 0.0011461991149902344}, {0.0061279, 0.0011125281860351562}, {0.0061512, 0.0011293255004882813}, {0.0061745, 0.0011085323242187501}, {0.0061978, 0.001096558868408203}, {0.0062211, 0.001115427587890625}, {0.0062444, 0.0010907770202636718}, {0.0062677, 0.001093679248046875}, {0.006291, 0.0010872050476074219}, {0.0063143, 0.001065405841064453}, {0.0063376000000000005, 0.0010893810119628907}, {0.0063609, 0.0010423773559570314}, {0.0063842000000000005, 0.0010539410522460938}, {0.0064075, 0.001061847998046875}, {0.0064308, 0.0010438411865234375}, {0.0064541, 0.0010391388427734374}, {0.0064774, 0.0010198688415527343}, {0.0065007, 0.000994749169921875}, {0.006524, 0.0010122049255371095}, {0.0065473, 0.000987311328125}, {0.0065706, 0.0010059115844726562}, {0.0065939, 0.000987483709716797}, {0.0066172, 0.0009742131530761719}, {0.006640500000000001, 0.0009791980895996093}, {0.0066638, 0.0009535217102050782}, {0.0066871000000000005, 0.0009643054504394531}, {0.0067104, 0.0009683126159667969}, {0.0067337000000000004, 0.0009328020080566407}, {0.006757, 0.0009595748474121094}, {0.0067803, 0.0009280968383789062}, {0.0068036, 0.0009304508361816406}, {0.0068269, 0.0009402285461425781}, {0.0068502, 0.0009117686279296875}, {0.0068735, 0.0009183869506835938}, {0.0068968, 0.0009000551574707031}, {0.0069201, 0.0008833341430664062}, {0.0069434, 0.0009059754760742187}, {0.0069667, 0.00085768037109375}, {0.0069900000000000006, 0.0008770294982910156}, {0.0070133, 0.0008552331176757813}, {0.0070366000000000005, 0.0008451417297363281}, {0.0070599, 0.0008462268859863281}, {0.0070832, 0.0008262390991210938}, {0.0071065, 0.0008383849365234375}, {0.0071298, 0.0008338210632324219}, {0.0071531, 0.0007974485473632813}, {0.0071764, 0.0008140000061035156}, {0.0071997, 0.0007814679260253906}, {0.007223, 0.000794809130859375}, {0.0072463, 0.0007862776550292969}, {0.0072696, 0.0007672082946777344}, {0.007292900000000001, 0.0007734253356933594}, {0.0073162, 0.0007566901916503906}, {0.0073395000000000005, 0.0007445019653320313}, {0.0073628, 0.0007607595275878907}, {0.0073861000000000005, 0.000750272509765625}, {0.0074094, 0.0007534629821777344}, {0.0074327, 0.0007220754028320313}, {0.007456, 0.0007098730468750001}, {0.0074793, 0.000714191064453125}, {0.0075026, 0.0006953788635253906}, {0.0075259, 0.0006995584106445313}, {0.0075492, 0.0006839112487792969}, {0.0075725, 0.0006730851196289063}, {0.0075958, 0.0006783950378417969}, {0.0076191, 0.0006461059875488281}, {0.007642400000000001, 0.000648991259765625}, {0.0076657, 0.0006598484741210937}, {0.0076890000000000005, 0.0006329541198730468}, {0.0077123, 0.0006504890014648437}, {0.0077356000000000005, 0.0006358959106445313}, {0.0077589, 0.0006347146728515625}, {0.0077822, 0.0006336266906738281}, {0.0078055, 0.0006184966735839843}, {0.0078288, 0.0006264347045898438}, {0.0078521, 0.0006099171569824219}, {0.0078754, 0.00059380654296875}, {0.0078987, 0.0006151762084960938}, {0.007922, 0.0005985597534179688}, {0.0079453, 0.0005993764465332031}, {0.007968600000000001, 0.0005692520568847656}, {0.0079919, 0.0005665250366210938}, {0.0080152, 0.000563037841796875}, {0.0080385, 0.0005617605224609375}, {0.008061800000000001, 0.0005631452270507813}, {0.0080851, 0.0005573181640625}, {0.0081084, 0.0005523756164550781}, {0.0081317, 0.0005436378479003907}, {0.008155, 0.0005400121826171875}, {0.0081783, 0.0005252551879882813}, {0.0082016, 0.0005320091552734375}, {0.0082249, 0.0005122926574707031}, {0.0082482, 0.0005191907470703125}, {0.0082715, 0.0005086076477050782}, {0.0082948, 0.00048188284912109374}, {0.0083181, 0.0004859041442871094}, {0.0083414, 0.000470618701171875}, {0.008364700000000001, 0.00047443370361328126}, {0.008388, 0.00047176602783203126}, {0.0084113, 0.00048058574829101564}, {0.0084346, 0.0004661904724121094}, {0.0084579, 0.0004479830200195313}, {0.0084812, 0.0004529086120605469}, {0.0085045, 0.00046597852783203126}, {0.0085278, 0.00045447135009765623}, {0.0085511, 0.0004456035888671875}, {0.0085744, 0.00042174428100585936}, {0.0085977, 0.00041809883422851563}, {0.008621, 0.00043411336669921876}, {0.0086443, 0.0004134417053222656}, {0.008667600000000001, 0.00041378929443359374}, {0.0086909, 0.000404333740234375}, {0.0087142, 0.00039026909790039065}, {0.0087375, 0.0004057043151855469}, {0.008760800000000001, 0.00039212008056640623}, {0.0087841, 0.000400490478515625}, {0.0088074, 0.0003791603759765625}, {0.0088307, 0.000370219140625}, {0.008854, 0.0003812261291503906}, {0.0088773, 0.00036329844360351565}, {0.0089006, 0.0003583389404296875}, {0.0089239, 0.000354733056640625}, {0.0089472, 0.00032796869506835936}, {0.008970500000000001, 0.0003393939208984375}, {0.0089938, 0.000331718701171875}, {0.0090171, 0.00033406139526367186}, {0.0090404, 0.00033278690185546873}, {0.009063700000000001, 0.00030019547729492186}, {0.009087, 0.00031821359252929687}, {0.0091103, 0.00031008905029296873}, {0.0091336, 0.0003061836181640625}, {0.0091569, 0.0002982540649414063}, {0.0091802, 0.0002736430603027344}, {0.0092035, 0.0002926559020996094}, {0.0092268, 0.00028394074096679687}, {0.0092501, 0.0002632690795898438}, {0.0092734, 0.00027260594482421874}, {0.0092967, 0.00026199176025390626}]}, {[{0.0, 0.0006931904781904768}, {2.33e-05, 0.0006994862924834821}, {4.66e-05, 0.0007058158662194502}, {6.99e-05, 0.0007121791165404568}, {9.32e-05, 0.0007185759530260135}, {0.0001165, 0.0007250062775080267}, {0.0001398, 0.0007314699838825174}, {0.0001631, 0.0007379669579180747}, {0.0001864, 0.0007444970770610205}, {0.0002097, 0.0007510602102372696}, {0.000233, 0.0007576562176508601}, {0.0002563, 0.0007642849505791454}, {0.0002796, 0.0007709462511646273}, {0.0003029, 0.0007776399522034235}, {0.0003262, 0.0007843658769303565}, {0.0003495, 0.0007911238388006612}, {0.0003728, 0.0007979136412683039}, {0.00039610000000000003, 0.0008047350775609155}, {0.0004194, 0.0008115879304513398}, {0.0004427, 0.0008184719720258032}, {0.000466, 0.0008253869634487166}, {0.0004893, 0.0008323326547241221}, {0.0005126, 0.0008393087844538029}, {0.0005359, 0.0008463150795920792}, {0.0005592, 0.0008533512551973149}, {0.0005825, 0.0008604170141801686}, {0.0006058, 0.0008675120470486245}, {0.0006291000000000001, 0.0008746360316498456}, {0.0006524, 0.0008817886329088959}, {0.0006757, 0.0008889695025643867}, {0.000699, 0.0008961782789011056}, {0.0007223, 0.0009034145864796945}, {0.0007456, 0.0009106780358634502}, {0.0007689, 0.000917968223342328}, {0.0007922000000000001, 0.0009252847306542362}, {0.0008155, 0.0009326271247037162}, {0.0008388, 0.0009399949572781144}, {0.0008621, 0.0009473877647613561}, {0.0008854, 0.0009548050678454448}, {0.0009087, 0.0009622463712398177}, {0.000932, 0.0009697111633786964}, {0.0009553000000000001, 0.0009771989161265874}, {0.0009786, 0.0009847090844820898}, {0.0010019, 0.0009922411062801865}, {0.0010252, 0.0009997944018932008}, {0.0010485, 0.0010073683739306152}, {0.0010718, 0.0010149624069379609}, {0.0010951000000000001, 0.0010225758670949993}, {0.0011184, 0.0010302081019134286}, {0.0011417, 0.001037858439934367}, {0.001165, 0.0010455261904258703}, {0.0011883, 0.0010532106430807655}, {0.0012116, 0.0010609110677150884}, {0.0012349, 0.0010686267139674362}, {0.0012582000000000001, 0.0010763568109995567}, {0.0012815, 0.0010841005671985153}, {0.0013048, 0.0010918571698807977}, {0.0013281, 0.0010996257849987183}, {0.0013514, 0.0011074055568495347}, {0.0013747, 0.001115195607787669}, {0.001398, 0.0011229950379404738}, {0.0014213000000000001, 0.0011308029249279844}, {0.0014446, 0.0011386183235871272}, {0.0014679, 0.0011464402657008718}, {0.0014912, 0.0011542677597328307}, {0.0015145, 0.001162099790567838}, {0.0015378, 0.001169935319259049}, {0.0015611, 0.0011777732827821334}, {0.0015844000000000001, 0.0011856125937971486}, {0.0016077, 0.0011934521404187003}, {0.001631, 0.0012012907859950278}, {0.0016543, 0.001209127368896655}, {0.0016776, 0.0012169607023152877}, {0.0017009, 0.001224789574073644}, {0.0017242, 0.0012326127464469328}, {0.0017475000000000001, 0.0012404289559967108}, {0.0017708, 0.0012482369134178715}, {0.0017941, 0.0012560353033995361}, {0.0018174, 0.0012638227845006348}, {0.0018407, 0.0012715979890409847}, {0.001864, 0.0012793595230086888}, {0.0018873, 0.0012871059659846917}, {0.0019106000000000001, 0.0012948358710853476}, {0.0019339000000000001, 0.001302547764923864}, {0.0019572, 0.001310240147591501}, {0.0019805, 0.001317911492659409}, {0.0020038, 0.001325560247202006}, {0.0020271, 0.001333184831842788}, {0.0020504, 0.0013407836408234855}, {0.0020737, 0.0013483550420974645}, {0.002097, 0.0013558973774482803}, {0.0021203, 0.0013634089626342852}, {0.0021436, 0.0013708880875601761}, {0.0021669000000000002, 0.0013783330164763724}, {0.0021902000000000002, 0.0013857419882070798}, {0.0022135, 0.0013931132164078965}, {0.0022368, 0.0014004448898537788}, {0.0022601, 0.0014077351727581654}, {0.0022834, 0.0014149822051240204}, {0.0023067, 0.0014221841031275204}, {0.00233, 0.0014293389595350639}, {0.0023533, 0.0014364448441542316}, {0.0023766, 0.0014434998043192683}, {0.0023999, 0.0014505018654115927}, {0.0024232, 0.0014574490314157686}, {0.0024465, 0.0014643392855112898}, {0.0024698, 0.0014711705907004438}, {0.0024931000000000003, 0.0014779408904724161}, {0.0025164000000000002, 0.0014846481095036903}, {0.0025397, 0.0014912901543946801}, {0.002563, 0.0014978649144423918}, {0.0025863, 0.0015043702624487755}, {0.0026096, 0.001510804055564261}, {0.0026329, 0.001517164136165801}, {0.0026562, 0.001523448332768551}, {0.0026795, 0.0015296544609701077}, {0.0027028, 0.0015357803244259946}, {0.0027261, 0.0015418237158548336}, {0.0027494, 0.0015477824180713585}, {0.0027727, 0.001553654205045126}, {0.002796, 0.001559436842982436}, {0.0028193000000000003, 0.0015651280914285982}, {0.0028426000000000002, 0.0015707257043872662}, {0.0028659000000000002, 0.0015762274314530956}, {0.0028892, 0.001581631018953456}, {0.0029125, 0.0015869342110943416}, {0.0029358, 0.0015921347511049621}, {0.0029591, 0.0015972303823747315}, {0.0029824, 0.001602218849575508}, {0.0030057, 0.0016070978997609349}, {0.003029, 0.0016118652834335738}, {0.0030523, 0.0016165187555691556}, {0.0030756, 0.0016210560765856773}, {0.0030989, 0.0016254750132431706}, {0.0031222, 0.00162977333945769}, {0.0031455, 0.001633948837010323}, {0.0031688000000000003, 0.0016379992961286696}, {0.0031921000000000002, 0.0016419225159141418}, {0.0032154, 0.0016457163045833128}, {0.0032387, 0.0016493784794851718}, {0.003262, 0.0016529068668480493}, {0.0032853, 0.0016562993011996258}, {0.0033086, 0.0016595536243900553}, {0.0033319, 0.0016626676841306836}, {0.0033552, 0.0016656393319375417}, {0.0033785, 0.0016684664203374042}, {0.0034018, 0.001671146799151227}, {0.0034251, 0.0016736783106099347}, {0.0034484, 0.0016760587829725134}, {0.0034717, 0.0016782860221929877}, {0.0034950000000000003, 0.0016803578009992881}, {0.0035183000000000002, 0.0016822718444661157}, {0.0035416, 0.0016840258107197758}, {0.0035649, 0.0016856172646834472}, {0.0035882, 0.0016870436415173176}, {0.0036115, 0.0016883021941302685}, {0.0036348, 0.0016893899147098295}, {0.0036581, 0.0016903034108135253}, {0.0036814, 0.001691038694128607}, {0.0037047, 0.001691590776774422}, {0.003728, 0.0016919527374693766}, {0.0037513, 0.0016921123980260522}, {0.0037746, 0.0016920390924644126}, {0.0037979, 0.0016917528929810167}, {0.0038212000000000003, 0.0016912729141044939}, {0.0038445000000000003, 0.0016906073886792169}, {0.0038678000000000002, 0.0016897618842632225}, {0.0038911, 0.0016887407087519393}, {0.0039144, 0.001687547451584867}, {0.0039377, 0.0016861852502939932}, {0.003961, 0.0016846569410040458}, {0.0039843000000000005, 0.0016829651512725314}, {0.0040076, 0.0016811123610195858}, {0.0040309000000000005, 0.0016791009443691384}, {0.0040542, 0.0016769331993750718}, {0.0040775, 0.0016746113696908948}, {0.0041008, 0.0016721376606752712}, {0.0041241, 0.001669514251532567}, {0.0041474, 0.0016667433045527201}, {0.0041707, 0.0016638269721811236}, {0.004194, 0.0016607674024338027}, {0.0042173, 0.0016575667430298586}, {0.0042406, 0.0016542271445153373}, {0.0042639, 0.0016507507625843373}, {0.0042872, 0.001647139759754485}, {0.0043105, 0.0016433963065185368}, {0.0043338000000000005, 0.001639522582067806}, {0.0043571, 0.0016355207746635576}, {0.0043804000000000004, 0.00163139308171769}, {0.0044037, 0.0016271417096326182}, {0.004427, 0.001622768873441378}, {0.0044503, 0.0016182767962820079}, {0.0044736, 0.0016136677087346884}, {0.0044969, 0.001608943848045669}, {0.0045202, 0.0016041074572583874}, {0.0045435, 0.0015991607842692338}, {0.0045668, 0.001594106080822949}, {0.0045901, 0.0015889456014606344}, {0.0046134, 0.0015836816024316193}, {0.0046367, 0.0015783163405790007}, {0.00466, 0.0015728520722074252}, {0.0046833000000000005, 0.0015672910519406336}, {0.0047066, 0.0015616355315753664}, {0.0047299, 0.0015558877589374263}, {0.0047532, 0.0015500499767450062}, {0.0047765, 0.0015441244214837626}, {0.0047998, 0.001538113322297575}, {0.0048231, 0.0015320188998984446}, {0.0048464, 0.0015258433654985481}, {0.0048697, 0.0015195889197670725}, {0.004893, 0.0015132577518141093}, {0.0049163, 0.0015068520382035546}, {0.0049396, 0.0015003739419966946}, {0.0049629, 0.0014938256118278666}, {0.0049862000000000005, 0.0014872091810133748}, {0.0050095, 0.0014805267666945974}, {0.0050328000000000005, 0.0014737804690160411}, {0.0050561, 0.0014669723703389125}, {0.0050794, 0.0014601045344906022}, {0.0051027, 0.001453179006050345}, {0.005126, 0.0014461978096711602}, {0.0051493, 0.0014391629494380734}, {0.0051726, 0.0014320764082624865}, {0.0051959, 0.0014249401473124782}, {0.0052192, 0.0014177561054787076}, {0.0052425, 0.001410526198875526}, {0.0052658, 0.001403252320376808}, {0.0052891, 0.0013959363391859644}, {0.0053124, 0.0013885801004395225}, {0.0053357000000000005, 0.001381185424843618}, {0.005359, 0.0013737541083426897}, {0.0053823000000000005, 0.001366287921819627}, {0.0054056, 0.0013587886108265923}, {0.0054289, 0.0013512578953456971}, {0.0054522, 0.0013436974695787006}, {0.0054755, 0.0013361090017648656}, {0.0054988, 0.0013284941340261022}, {0.0055221, 0.0013208544822385024}, {0.0055454, 0.001313191635929379}, {0.0055687, 0.0013055071581988956}, {0.005592, 0.0012978025856653897}, {0.0056153, 0.0012900794284334768}, {0.0056386000000000006, 0.0012823391700840419}, {0.0056619, 0.0012745832676852105}, {0.0056852000000000005, 0.001266813151823414}, {0.0057085, 0.001259030226653672}, {0.0057318000000000004, 0.0012512358699682104}, {0.0057551, 0.0012434314332825712}, {0.0057784, 0.0012356182419383547}, {0.0058017, 0.001227797595221782}, {0.005825, 0.0012199707664972464}, {0.0058483, 0.001212139003355078}, {0.0058716, 0.0012043035277727238}, {0.0058949, 0.001196465536288602}, {0.0059182, 0.0011886262001878764}, {0.0059415, 0.0011807866656994433}, {0.0059648, 0.0011729480542034176}, {0.0059881000000000005, 0.0011651114624484525}, {0.0060114, 0.0011572779627782223}, {0.0060347000000000005, 0.0011494486033664356}, {0.006058, 0.0011416244084597631}, {0.0060813, 0.001133806378628077}, {0.0061046, 0.0011259954910214337}, {0.0061279, 0.0011181926996332366}, {0.0061512, 0.001110398935569054}, {0.0061745, 0.0011026151073205662}, {0.0061978, 0.001094842101044159}, {0.0062211, 0.0010870807808436777}, {0.0062444, 0.0010793319890568958}, {0.0062677, 0.0010715965465452554}, {0.006291, 0.0010638752529864666}, {0.0063143, 0.0010561688871695625}, {0.0063376000000000005, 0.0010484782072920328}, {0.0063609, 0.0010408039512586685}, {0.0063842000000000005, 0.0010331468369817727}, {0.0064075, 0.00102550756268241}, {0.0064308, 0.0010178868071923735}, {0.0064541, 0.0010102852302565826}, {0.0064774, 0.001002703472835615}, {0.0065007, 0.00099514215740812}, {0.006524, 0.000987601888272844}, {0.0065473, 0.0009800832518500433}, {0.0065706, 0.0009725868169820455}, {0.0065939, 0.0009651131352327557}, {0.0066172, 0.0009576627411859001}, {0.006640500000000001, 0.0009502361527418221}, {0.0066638, 0.0009428338714126536}, {0.0066871000000000005, 0.0009354563826156915}, {0.0067104, 0.0009281041559648328}, {0.0067337000000000004, 0.0009207776455599127}, {0.006757, 0.000913477290273823}, {0.0067803, 0.0009062035140372727}, {0.0068036, 0.0008989567261210874}, {0.0068269, 0.0008917373214159297}, {0.0068502, 0.0008845456807093494}, {0.0068735, 0.0008773821709600665}, {0.0068968, 0.0008702471455694099}, {0.0069201, 0.0008631409446498288}, {0.0069434, 0.0008560638952904167}, {0.0069667, 0.000849016311819375}, {0.0069900000000000006, 0.000841998496063372}, {0.0070133, 0.0008350107376037375}, {0.0070366000000000005, 0.0008280533140294542}, {0.0070599, 0.0008211264911869073}, {0.0070832, 0.0008142305234263548}, {0.0071065, 0.0008073656538450969}, {0.0071298, 0.0008005321145273117}, {0.0071531, 0.0007937301267805472}, {0.0071764, 0.0007869599013688453}, {0.0071997, 0.0007802216387424953}, {0.007223, 0.0007735155292644008}, {0.0072463, 0.0007668417534330638}, {0.0072696, 0.0007602004821021775}, {0.007292900000000001, 0.0007535918766968387}, {0.0073162, 0.000747016089426377}, {0.0073395000000000005, 0.0007404732634938137}, {0.0073628, 0.0007339635333019611}, {0.0073861000000000005, 0.0007274870246561715}, {0.0074094, 0.0007210438549637572}, {0.0074327, 0.0007146341334300921}, {0.007456, 0.0007082579612514207}, {0.0074793, 0.0007019154318043912}, {0.0075026, 0.0006956066308323387}, {0.0075259, 0.0006893316366283405}, {0.0075492, 0.0006830905202150725}, {0.0075725, 0.000676883345521491}, {0.0075958, 0.0006707101695563709}, {0.0076191, 0.0006645710425787287}, {0.007642400000000001, 0.0006584660082651626}, {0.0076657, 0.0006523951038741387}, {0.0076890000000000005, 0.0006463583604072591}, {0.0077123, 0.0006403558027675442}, {0.0077356000000000005, 0.0006343874499147606}, {0.0077589, 0.0006284533150178359}, {0.0077822, 0.0006225534056043864}, {0.0078055, 0.0006166877237074037}, {0.0078288, 0.0006108562660091267}, {0.0078521, 0.000605059023982144}, {0.0078754, 0.0005992959840277572}, {0.0078987, 0.0005935671276116445}, {0.007922, 0.0005878724313968648}, {0.0079453, 0.000582211867374234}, {0.007968600000000001, 0.0005765854029901161}, {0.0079919, 0.0005709930012716638}, {0.0080152, 0.0005654346209495463}, {0.0080385, 0.0005599102165782063}, {0.008061800000000001, 0.0005544197386536765}, {0.0080851, 0.0005489631337289997}, {0.0081084, 0.0005435403445272843}, {0.0081317, 0.0005381513100524395}, {0.008155, 0.0005327959656976197}, {0.0081783, 0.0005274742433514206}, {0.0082016, 0.0005221860715018592}, {0.0082249, 0.0005169313753381807}, {0.0082482, 0.0005117100768505208}, {0.0082715, 0.0005065220949274651}, {0.0082948, 0.0005013673454515367}, {0.0083181, 0.0004962457413926547}, {0.0083414, 0.0004911571928995887}, {0.008364700000000001, 0.00048610160738945195}, {0.008388, 0.0004810788896352649}, {0.0084113, 0.00047608894185162013}, {0.0084346, 0.00047113166377849025}, {0.0084579, 0.0004662069527632024}, {0.0084812, 0.00046131470384061935}, {0.0085045, 0.0004564548098115553}, {0.0085278, 0.00045162716131946394}, {0.0085511, 0.0004468316469254234}, {0.0085744, 0.00044206815318145526}, {0.0085977, 0.00043733656470220446}, {0.008621, 0.00043263676423501557}, {0.0086443, 0.00042796863272842947}, {0.008667600000000001, 0.00042333204939913453}, {0.0086909, 0.0004187268917974002}, {0.0087142, 0.0004141530358710204}, {0.0087375, 0.0004096103560277995}, {0.008760800000000001, 0.00040509872519660313}, {0.0087841, 0.0004006180148870056}, {0.0088074, 0.0003961680952475583}, {0.0088307, 0.0003917488351227105}, {0.008854, 0.00038736010210840225}, {0.0088773, 0.00038300176260636077}, {0.0089006, 0.00037867368187712204}, {0.0089239, 0.00037437572409180743}, {0.0089472, 0.00037010775238267423}, {0.008970500000000001, 0.0003658696288924687}, {0.0089938, 0.00036166121482260414}, {0.0090171, 0.0003574823704801859}, {0.0090404, 0.00035333295532391116}, {0.009063700000000001, 0.0003492128280088599}, {0.009087, 0.0003451218464302042}, {0.0091103, 0.00034105986776585446}, {0.0091336, 0.00033702674851806874}, {0.0091569, 0.00033302234455404045}, {0.0091802, 0.00032904651114548964}, {0.0092035, 0.00032509910300727553}, {0.0092268, 0.0003211799743350542}, {0.0092501, 0.000317288978841996}, {0.0092734, 0.0003134259697945863}, {0.0092967, 0.00030959080004752524}]}]
  # "Captures a background image and subtracts this file from continuously captured images (always takes logarithm)."
  # "PixelFly Camera Controls"
  # "Software Image Manipulation"
  # "Experimental Parameters"
  # "Analog  Voltage Monitors"
  # "PixelFly full image area is 1024 in columns and 1280 in rows.\nIndex starts at 1."
  # "2D fitting"
  # "1D fitting"
  # "Applies to 1D arbitrary fit."
  # "ROI is applied\nbefore binning"
  # "Applies to 1D fit."
  # "Form a matrix using only one point for every\nsampleinterleave points in a row/column."
  # "Files only saved when \"continuous\" is turned off. MAke sure that you use .dat xtension when saving as asci and .bny when saving as binary. Yo select format in back panel."
  # "Applies to 1D arbitrary fit."
  # "Number of columns and rows at the\ncorners to find uncertainties/noise."
  # "Number of pixels in smoothing\nfor plotting residuals."
  # "Isotope"
  # "Avg. Temp (uK)"
  # "Drop Time (ms)"
  # "<-------- toward source <----------"
  # "<-------- toward source <----------"
  # "gravity\n  |\n  |\n  |\n  V"
  # "MAXIMUM COUNTS FOR PIXELFLY \nSINGLE SHOT: 4096"
  # "gravity\n  |\n  |\n  |\n  V"
  # "<-------- toward source <----------"
  # "2D Fitting"
  # "1D Fitting"
  # "x                  y"
  # "Camera Indicators\nto Ignore"
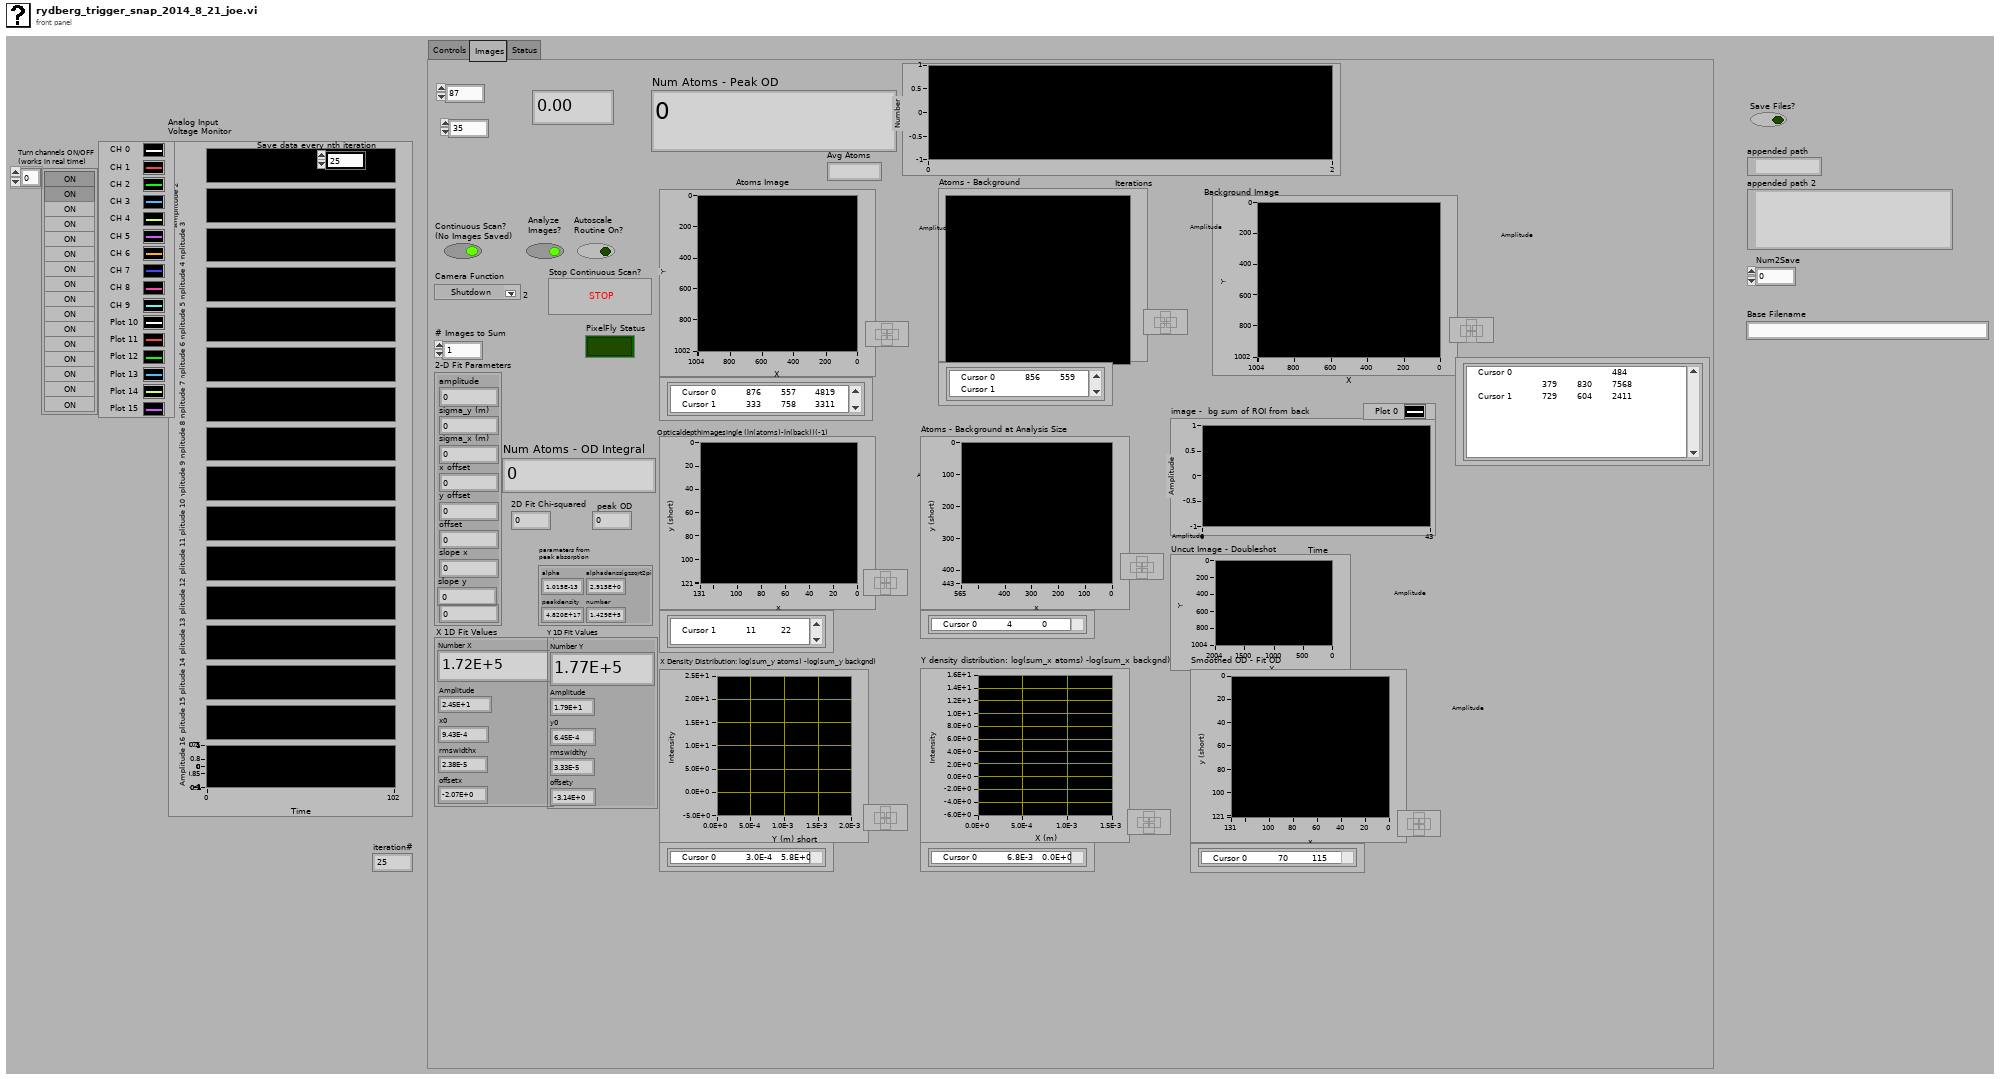
[diagram p1: front panel]
types:
  T1 = cluster{"data[0]":dbl, "data[1]":dbl, "data[2]":dbl, "data[3]":dbl, "data[4]":dbl, "data[5]":dbl, "data[6]":dbl, "data[7]":dbl, "data[8]":dbl, "data[9]":dbl, "data[10]":dbl, "data[11]":dbl, "data[12]":dbl, "data[13]":dbl, "data[14]":dbl, "data[15]":dbl}
  T2 = cluster{"Col Start":i32, "Col Stop":i32, "Row Start":i32, "Row stop":i32}
  T3 = typedef "camera_controls.ctl" = cluster{"Acquisition Mode":T4, "Trigger Mode":T5, "Frame \nTransfer":bool, "Exposure Time (s)":sgl, "Accumulation Cycle Time (s)":sgl, "# Accumulations":i32, "# Kinetics":i32, "Kinetic Cycle Time (s)":sgl, "Horizontal Bin Size":i32, "Vertical Bin Size":i32}
  T4 = typedef "AcquisitionMode_mode typedef.ctl" = enum16{"Reserved (0)", "Single Scan", "Accumulate", "Kinetics", "Fast Kinetics", "Run Till Abort", "Reserved (6)", "Reserved (7)", "Reserved (8)", "Time Delayed Integration"}
  T5 = typedef "TriggerMode_mode typedef.ctl" = enum16{"Internal", "External", "N/A (2)", "N/A (3)", "N/A (4)", "N/A (5)", "External Start", "External Exposure (Bulb)", "N/A (8)", "External FVB EM", "Software", "N/A (11)", "External Charge Shifting"}
  T6 = cluster{"alpha":dbl, "peakdensity":dbl, "alphadenssigzsqrt2pi":sgl, "number":dbl}
  T7 = cluster{"Amplitude":dbl, "y0":dbl, "rmswidthy":dbl, "offsety":dbl, "Number Y":dbl}
  T8 = cluster{"Amplitude":dbl, "x0":dbl, "rmswidthx":dbl, "offsetx":dbl, "Number X":dbl}
  T9 = cluster{"amplitude":dbl, "sigma_y (m)":dbl, "sigma_x (m)":dbl, "x offset":dbl, "y offset":dbl, "offset":dbl, "slope x":dbl, "slope y":dbl, dbl}
  T10 = cluster{"xpixels":i32, "ypixels":i32, "# VS Speeds":i32, "VS Speed (us)":sgl, "Temperature Stable":bool, "Temperature (C)":i32}
  T11 = cluster{"amplitudey":dbl, "temperaturey":dbl, "alphay":dbl, "offsety":dbl, "numbery":dbl, "peakdensityy":dbl, "centery":dbl}
  T12 = cluster{"amplitudex":dbl, "temperaturex":dbl, "alphax":dbl, "offsetx":dbl, "numberx":dbl, "peakdensityx":dbl, "centerx":dbl}
  T13 = cluster{"Initalize Error Code":u32, "GetDetector Error Code":u32, "Get#VSSpeeds Error Code":u32, "Set VS Speed Error":u32, "CoolerOn Error Code":u32, "GetTemperature Error Code":u32, "Shutdown Error Code":u32}
  T14 = cluster{"Sample Interleave":dbl, "Pixel Size (m)":dbl, i32, "Cut Borders":dbl, "Number for Scale":dbl, "Limit":dbl, "Number of Pixels to Smooth":dbl}
  T15 = typedef "LVCursorListTypeDef.ctl" = cluster{"Name":string, "Color":u32, "Style":u8, "Point Style":u8, "Name Visible":bool, "Allow Drag":bool, "Cursor Mode":u32, "Plot":i32, "Index":i32, "Position":cluster{"X":dbl, "Y":dbl}, "X Scale":u32, "Y Scale":u32, "Watch Plots":i32[], "Watch All Plots":bool, "Plot Area":i32, "Label Offset":cluster{"X":dbl, "Y":dbl}}[]
  T16 = cluster{"abscrosssection":dbl, "peakdensity":dbl, "twosizeoneoverezabsxsecdens":dbl, "number":dbl}
  T17 = cluster{"Amplitude":dbl, "x0":dbl, "rmswidthx":dbl, "offsetx":dbl, "numberx":dbl}
  T18 = cluster{"Amplitude":dbl, "y0":dbl, "rmswidthy":dbl, "offsety":dbl, "numbery":dbl}
  T19 = cluster{"amplitude":dbl, "sigma_y (m)":dbl, "sigma_x (m)":dbl, "row offset (pixel #)":dbl, "col offset (pixel #)":dbl, "offset":dbl, "slope x":dbl, "slope y":dbl, dbl}
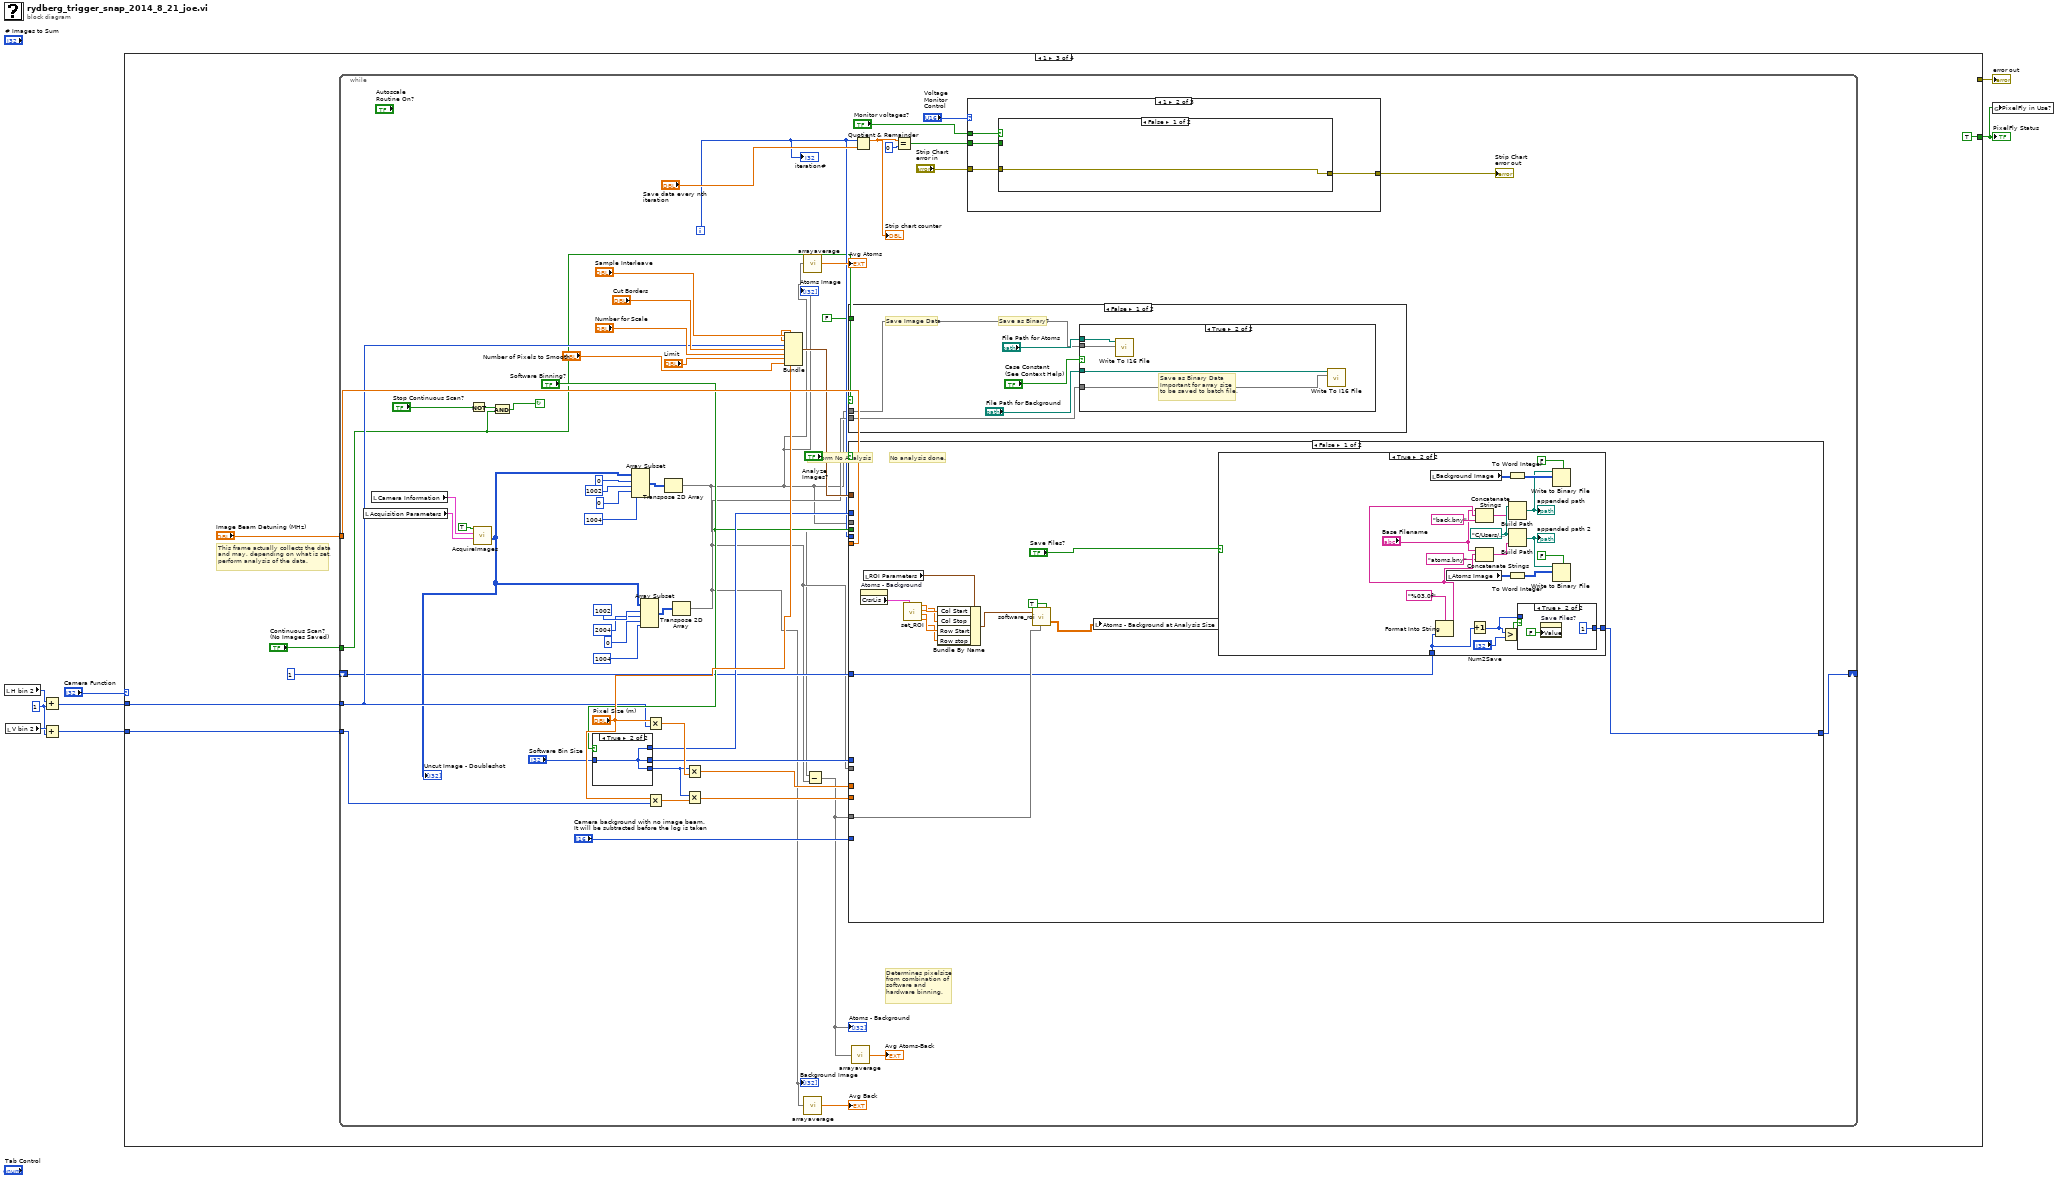
[diagram p0: block diagram]
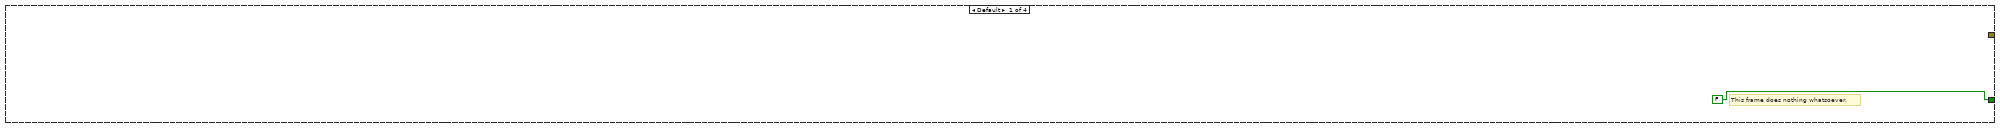
[diagram p2: hidden frame]
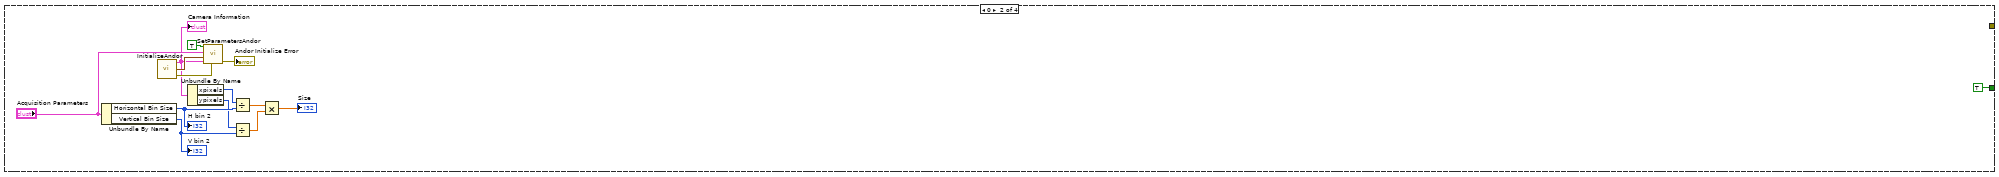
[diagram p3: hidden frame]
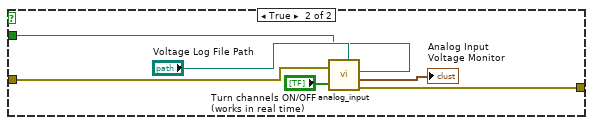
[diagram p5: hidden frame]
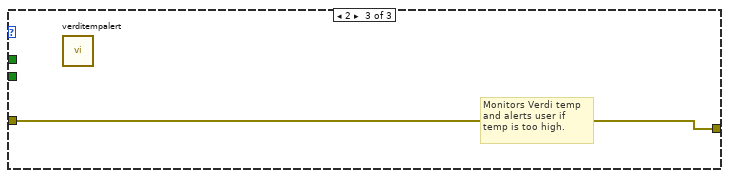
[diagram p6: hidden frame]
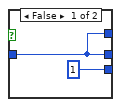
[diagram p7: hidden frame]
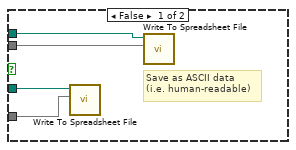
[diagram p8: hidden frame]
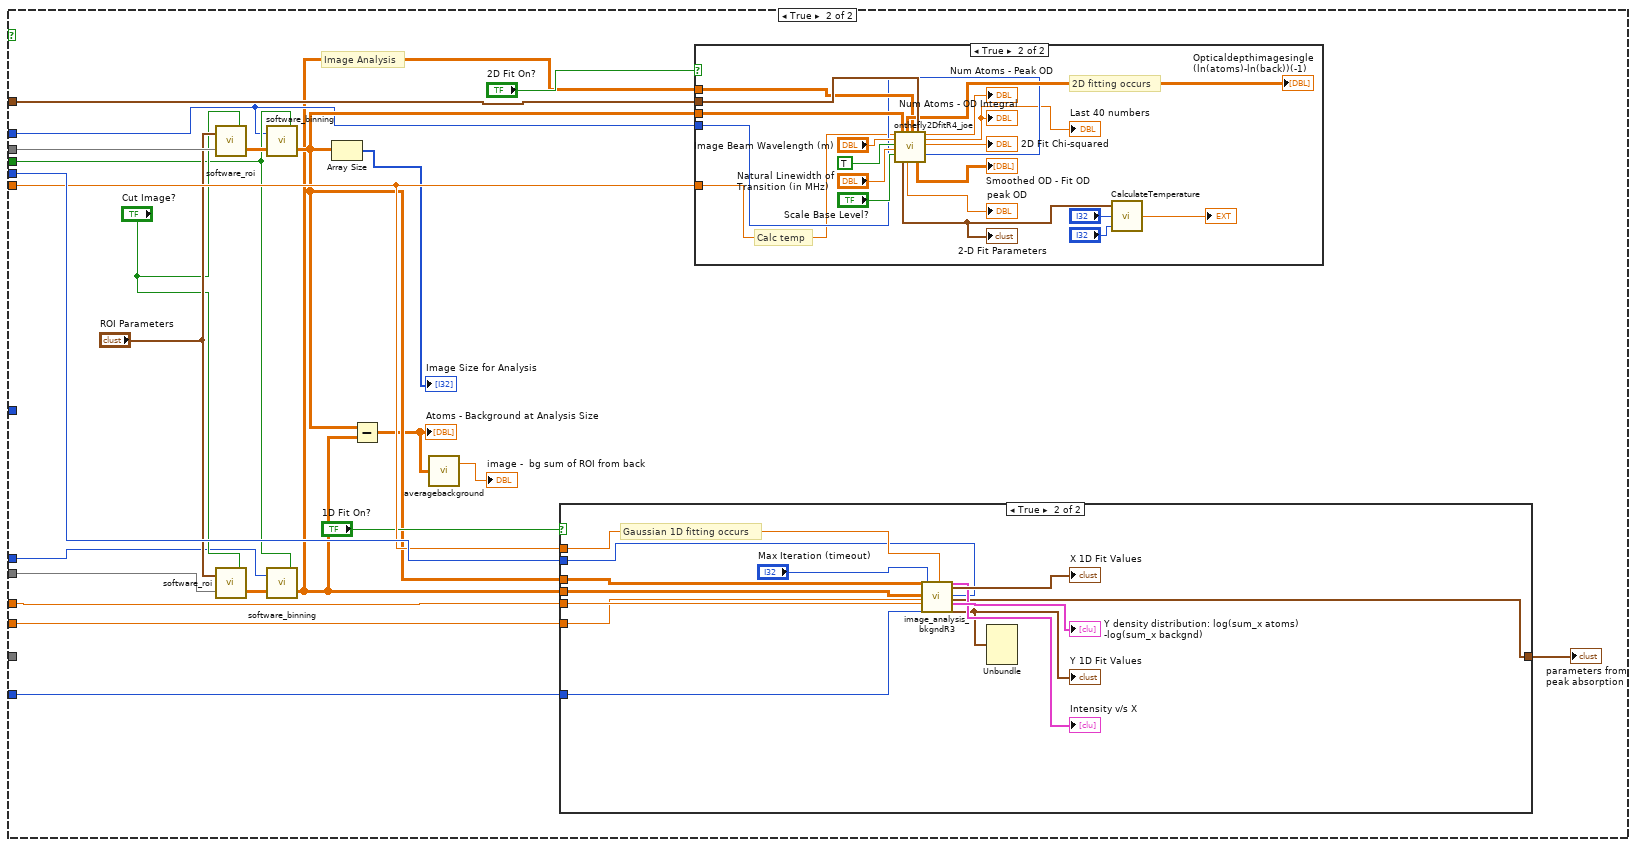
[diagram p12: hidden frame]
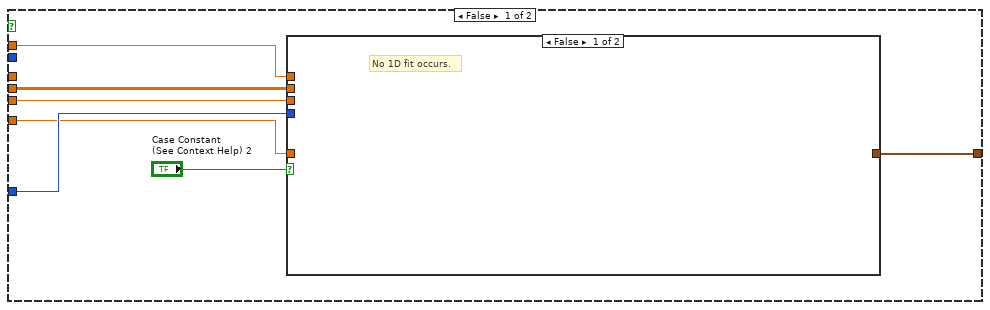
[diagram p14: hidden frame]
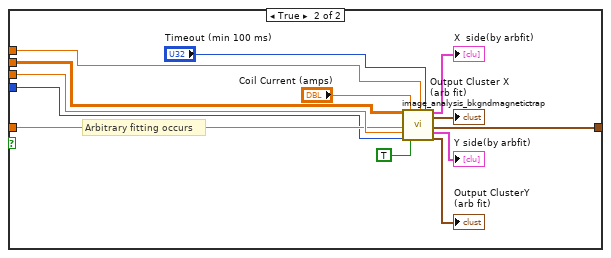
[diagram p15: hidden frame]
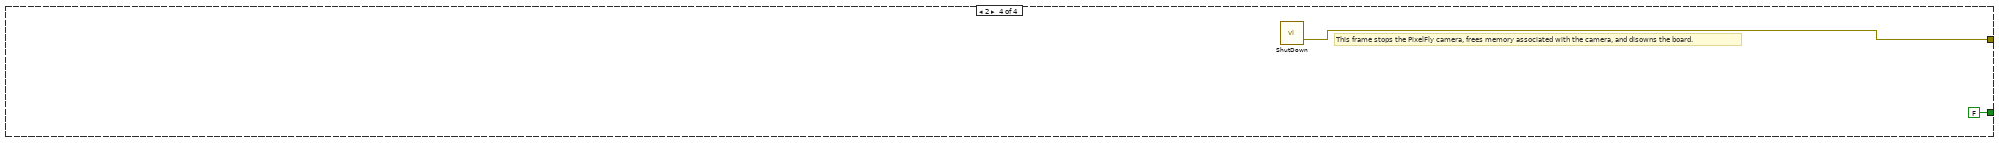
[diagram p16: hidden frame]
diagram:
  w3 = 1
  n1 = local read "H bin 2"() -> (w6:i32)
  n2 = local read "V bin 2"() -> (w4:i32)
  n3 = Add(x=w6, y=w3) -> (x+y=w5:i32)
  n4 = Add(x=w4, y=w3) -> (x+y=w2:i32)
  n5 = case shown="1" "Camera Function" {
    tunnel: w5 -> [_ _ w26 _]
    tunnel: w2 -> [_ _ w27 _]
    tunnel: [_ _ _ w228] -> w7
    tunnel: [FALSE TRUE TRUE FALSE] -> w1
    frame Default {
      # "This frame does nothing whatsoever."
    }
    frame 0 {
      n6 = Unbundle By Name("Acquisition Parameters") -> ("Horizontal Bin Size"=w15:i32, "Vertical Bin Size"=w13:i32)
      "H bin 2" <- w15
      "V bin 2" <- w13
      n7 = call "InitializeAndor.vi"() -> ("error out"=w22:errorcluster, "Andor Initialization Error Codes"=w21:T13, "Camera Information"=w17:T10)  [unwired: 3 in]
      "Camera Information" <- w17
      n8 = Unbundle By Name(w17) -> ("xpixels"=w16:i32, "ypixels"=w14:i32)
      n9 = call "SetParametersAndor.vi"("Error In"=w22, "Camera Information"=w17, "Andor Initialization Error Codes"=w21, "Acquisition Parameters"="Acquisition Parameters", "Pre Initialized?"=TRUE) -> ("error out"=→"Andor Initialize Error":errorcluster)  [unwired: 4 in, 2 out]
      n10 = Divide(x=w16, y=w15) -> (x/y=w11:dbl)
      n11 = Divide(x=w14, y=w13) -> (x/y=w12:dbl)
      n12 = Multiply(x=w11, y=w12) -> (x*y=→"Size":dbl)
    }
    frame 1 {
      # "This frame actually collects the data\nand may, depending on what is set,\nperform analysis of the data."
      n13 = while {
        tunnel: "Image Beam Detuning (MHz)" -> [w86]
        tunnel: "Continuous Scan?\n(No Images Saved)" -> [w49]
        tunnel: w27 -> [w82]
        tunnel: w26 -> [w53]
        shift-right: [w34] -> _
        shift-left: 1 -> [w35]
        i -> [w54]
        stop <- w85 continue-if-true
        # "Determines pixelsize\nfrom combination of\nsoftware and\nhardware binning."
        n14 = local read "Acquisition Parameters"() -> (w47:T3)
        n15 = local read "Camera Information"() -> (w46:T10)
        n16 = Not(x="Stop Continuous Scan?") -> (.not. x?=w83:bool)
        n17 = call "AcquireImages.vi"("Acquisition Parameters"=w47, "Camera Information 2"=w46, "Pre Initialized?"=TRUE) -> ("Intensity Graph"=w36:i32[][])  [unwired: 7 in, 1 out]
        "Uncut Image - Doubleshot" <- w36
        n18 = And(x=w83, y=w49) -> (x .and. y?=w85:bool)
        n19 = case shown="True" "Software Binning?" {
          tunnel: [w101 w102] -> w65
          tunnel: "Software Bin Size" -> [w101 w102]
          tunnel: [w101 w102] -> w63
          tunnel: [1 w102] -> w62
          frame False {
          }
          frame True {
          }
        }
        n20 = Array Subset(array=w36, index (row)=0, length (row)=1002 ("length"), index (col)=0 ("index"), length (col)=1004 ("length")) -> (w31:i32[][])
        n21 = Array Subset(array=w36, index (row)=1002, length (row)=2004 ("length"), index (col)=0 ("index"), length (col)=1004 ("length")) -> (w33:i32[][])
        n22 = Multiply(x="Pixel Size (m)", y=w53) -> (x*y=w76:dbl)
        n23 = Multiply(x="Pixel Size (m)", y=w82) -> (x*y=w75:dbl)
        n24 = Transpose 2D Array(2D array=w31) -> (transposed array=w30:i32[][])
        "Atoms Image" <- w30
        n25 = Transpose 2D Array(2D array=w33) -> (transposed array=w32:i32[][])
        "Background Image" <- w32
        n26 = Multiply(x=w62, y=w76) -> (x*y=w72:dbl)
        n27 = Multiply(x=w62, y=w75) -> (x*y=w74:dbl)
        n28 = Bundle("Sample Interleave"="Sample Interleave", "Pixel Size (m)"="Pixel Size (m)", w53, "Cut Borders"="Cut Borders", "Number for Scale"="Number for Scale", "Limit"="Limit", "Number of Pixels to Smooth"="Number of Pixels to Smooth") -> (w73:T14)  [unwired: 1 in]
        n29 = call "arrayaverage.vi"("Array int 32"=w30) -> ("Average"=→"Avg Atoms":ext)
        n30 = call "arrayaverage.vi"("Array int 32"=w32) -> ("Average"=→"Avg Back":ext)
        n31 = Subtract(x=w30, y=w32) -> (x-y=w37:i32[][])
        "Atoms - Background" <- w37
        n32 = case shown="False" w49 {
          tunnel: w30 -> [w104 _]
          tunnel: w32 -> [w103 _]
          tunnel: FALSE -> [_ _]
          frame False {
            # "Save as Binary?"
            # "Save Image Data"
            n33 = case shown="True" "Case Constant\n(See Context Help)" {
              tunnel: "File Path for Atoms" -> [w111 w115]
              tunnel: "File Path for Background" -> [w110 w114]
              tunnel: w104 -> [w109 w112]
              tunnel: w103 -> [w108 w113]
              frame False {
                # "Save as ASCII data\n(i.e. human-readable)"
                n34 = call-poly <vilib>:"Write To Spreadsheet File.vi"("2D data"=w108, "file path (dialog if empty)"=w110) -> ()  [unwired: 6 in, 1 out]
                n35 = call-poly <vilib>:"Write To Spreadsheet File.vi"("2D data"=w109, "file path (dialog if empty)"=w111) -> ()  [unwired: 6 in, 1 out]
              }
              frame True {
                # "Save as Binary Data\nImportant for array size\nto be saved to batch file."
                n36 = call <vilib>:"Write To I16 File.vi"("2D array"=w112, "file path (dialog if empty)"=w115) -> ()  [unwired: 5 in, 1 out]
                n37 = call <vilib>:"Write To I16 File.vi"("2D array"=w113, "file path (dialog if empty)"=w114) -> ()  [unwired: 5 in, 1 out]
              }
            }
          }
          frame True {
            # "Don't Save Data\nWhen Continous"
          }
        }
        n38 = case shown="False" "Analyze \nImages?" {
          tunnel: w72 -> [_ w165]
          tunnel: w74 -> [_ w164]
          tunnel: "Camera background with no image beam.\nIt will be subtracted before the log is taken" -> [_ w175]
          tunnel: w86 -> [_ w173]
          tunnel: w54 -> [_ w174]
          tunnel: w73 -> [_ w172]
          tunnel: w30 -> [_ w169]
          tunnel: w32 -> [_ w166]
          tunnel: w63 -> [_ w157]
          tunnel: "Software Binning?" -> [_ w160]
          tunnel: w65 -> [_ w159]
          tunnel: w37 -> [w128 _]
          tunnel: w35 -> [w125 _]
          tunnel: [w123 _] -> w34
          frame False {
            # "Perform No Analysis"
            # "No analysis done."
            n39 = property on="Atoms - Background" class="IntGraph (strict)"() -> ("CrsrLis"=w122:T15)  [unwired: 2 in, 2 out]
            n40 = local read "ROI Parameters"() -> (w121:T2)
            n41 = call "set_ROI.vi"("Cursor List"=w122) -> ("Row End"=w117:dbl, "RowStart"=w118:dbl, "ColEnd"=w119:dbl, "ColStart"=w120:dbl)  [unwired: 7 in]
            n42 = Bundle By Name(cluster=w121, "Col Start"=w120, "Col Stop"=w119, "Row Start"=w118, "Row stop"=w117) -> (w116:T2)
            n43 = call "software_roi.vi"("Cut image?"=TRUE, "Input Array"=w128, "ROI Controls"=w116) -> ("output array"=w127:sgl[][])
            n44 = local write "Atoms - Background at Analysis Size"(w127) -> ()
            n45 = case shown="True" "Save Files?" {
              tunnel: w125 -> [_ w133]
              tunnel: [_ w130] -> w123
              frame False {
              }
              frame True {
                w143 = path "C:/Users/Rydberg/Desktop/JoeDesktopFiles/Data and Analysis/Raw_Data/Sr88/2014.08.28" ("base path")
                n46 = local read "Background Image"() -> (w145:i32[][])
                n47 = Format Into String(format string="%03.0f", w133) -> (resulting string=w141:string)  [unwired: 2 in, 1 out]
                n48 = local read "Atoms Image"() -> (w147:i32[][])
                n49 = Increment(x=w133) -> (x+1=w129:i32)
                n50 = Concatenate Strings("Base Filename", w141, "back.bny" ("string")) -> (w138:string)
                n51 = Concatenate Strings("Base Filename", w141, "atoms.bny" ("string")) -> (w137:string)
                n52 = Greater?(x=w129, y="Num2Save") -> (0:w131:bool)
                n53 = To Word Integer(number=w145) -> (16bit integer=w144:i16[][])
                n54 = To Word Integer(number=w147) -> (16bit integer=w146:i16[][])
                n55 = Build Path(base path=w143, name or relative path=w138) -> (appended path=w135:path)
                "appended path" <- w135
                n56 = Build Path(base path=w143, name or relative path=w137) -> (appended path=w136:path)
                "appended path 2" <- w136
                n57 = case shown="True" w131 {
                  tunnel: [w150 1] -> w130
                  tunnel: w129 -> [w150 _]
                  frame False {
                  }
                  frame True {
                    n58 = property on="Save Files?" class="Bool (strict)"("Value"=FALSE ("Save Files?")) -> ()  [unwired: 2 in, 2 out]
                  }
                }
                n59 = Write to Binary File(file (use dialog)=w135, data=w144, 5:FALSE ("append to file? (new file:F)")) -> ()  [unwired: 3 in, 3 out]
                n60 = Write to Binary File(file (use dialog)=w136, data=w146, 5:FALSE ("append to file? (new file:F)")) -> ()  [unwired: 3 in, 3 out]
              }
            }
          }
          frame True {
            # "Image Analysis"
            n61 = call "software_roi.vi"("Cut image?"="Cut Image?", "Input Array"=w169, "ROI Controls"="ROI Parameters") -> ("output array"=w162:sgl[][])
            n62 = call "software_roi.vi"("Cut image?"="Cut Image?", "Input Array"=w166, "ROI Controls"="ROI Parameters") -> ("output array"=w161:sgl[][])
            n63 = call "software_binning.vi"("Bin image?"=w160, "Input Array"=w162, "bin size"=w157) -> ("Binned Array"=w158:dbl[][])
            n64 = call "software_binning.vi"("Bin image?"=w160, "Input Array"=w161, "bin size"=w159) -> ("Binned Array"=w156:dbl[][])
            n65 = Array Size(array=w158) -> (size(s)=→"Image Size for Analysis":i32[])
            n66 = Subtract(x=w158, y=w156) -> (x-y=w155:dbl[][])
            "Atoms - Background at Analysis Size" <- w155
            n67 = call "averagebackground.vi"("Input Array"=w155) -> ("sum of Gaussian"=→"image -  bg sum of ROI from back":dbl)  [unwired: 1 out]
            n68 = case shown="True" "1D Fit On?" {
              tunnel: w156 -> [w199 w217]
              tunnel: w175 -> [w201 w222]
              tunnel: w173 -> [w200 w226]
              tunnel: w158 -> [_ w218]
              tunnel: w174 -> [_ w221]
              tunnel: w165 -> [w197 w220]
              tunnel: w164 -> [w196 w219]
              tunnel: [w195 w215] -> w153
              frame False {
                n69 = case shown="False" "Case Constant\n(See Context Help) 2" {
                  tunnel: w197 -> [_ w213]
                  tunnel: w196 -> [_ w212]
                  tunnel: w201 -> [_ w211]
                  tunnel: w200 -> [_ w209]
                  tunnel: w199 -> [_ w204]
                  tunnel: [_ w202] -> w195
                  frame False {
                    # "No 1D fit occurs."
                  }
                  frame True {
                    # "Arbitrary fitting occurs"
                    n70 = call "image_analysis_bkgndmagnetictrap.vi"("2D Array In"=w204, "Delta_x (m)"=w212, "Delta_y (m)"=w213, "camera background with no image beam\nIt will be subtracted before the log is taken"=w211, "coilcurrent"="Coil Current (amps)", "take new\nnew image"=TRUE ("take new\nnew image"), "Image beam \nDetuning (MHz)"=w209, "timeout(min 100ms)"="Timeout (min 100 ms)") -> ("X  side"=→"X  side(by arbfit)":cluster{cluster{dbl, dbl}[]}[], "Output Cluster X"=→"Output Cluster X\n(arb fit)":T12, "parameters from\n peak absorption"=w202:T16, "Y side"=→"Y side(by arbfit)":cluster{cluster{dbl, dbl}[]}[], "Output ClusterY"=→"Output ClusterY\n(arb fit)":T11)  [unwired: 5 in, 2 out]
                  }
                }
              }
              frame True {
                # "Gaussian 1D fitting occurs"
                n71 = call "image_analysis_bkgndR3.vi"("Atoms array in"=w218, "BG array in"=w217, "Delta_x (m)"=w219, "Delta_y (m)"=w220, "camera background with no image beam\nIt will be subtracted before the log is taken"=w222, "max iteration"="Max Iteration (timeout)", "Image beam \nDetuning (MHz)"=w226, "Iteration #"=w221) -> ("Intensity v/s X 2"=→"Intensity v/s X":cluster{dbl[], dbl[]}[], "x fit values"=→"X 1D Fit Values":T17, "parameters from \npeak absorption"=w215:T6, "Intensity v/s X"=→"Y density distribution: log(sum_x atoms) -log(sum_x backgnd)":cluster{dbl[], dbl[]}[], "y fit values"=w216:T18)  [unwired: 13 in, 2 out]
                "Y 1D Fit Values" <- w216
                n72 = Unbundle(w216) -> ()  [unwired: 5 out]
              }
            }
            "parameters from \npeak absorption" <- w153
            n73 = case shown="True" "2D Fit On?" {
              tunnel: w158 -> [_ w184]
              tunnel: w173 -> [_ w180]
              tunnel: w172 -> [_ w189]
              tunnel: w156 -> [_ w183]
              tunnel: w157 -> [_ w182]
              frame False {
                # "No 2D fitting occurs"
              }
              frame True {
                # "Calc temp"
                # "2D fitting occurs"
                n74 = call "onthefly2DfitR4_joe.vi"("Detuning in MHz"=w180, "Wavelength (m)"="Image Beam Wavelength (m)", "pass image method"=TRUE, "Natural Linewidth of Transition\n(ion fwhm in MHz)"="Natural Linewidth of Transition (in MHz)", "Scale Base Level?"="Scale Base Level?", "Atoms"=w184, "Background"=w183, "Specifics of Fitting Routines"=w189, "Software bin size"=w182) -> ("2-D Gaussian Fit Parameters"=w176:T19, "opticaldepthimagesingle\n(ln(atoms)-ln(back))(-1)"=→"Opticaldepthimagesingle (ln(atoms)-ln(back))(-1)":dbl[][], "peak OD"=→"peak OD":dbl, "smoothed OD-fit OD"=→"Smoothed OD - Fit OD":dbl[][], "# atoms from peakOD"=→"Num Atoms - Peak OD":dbl, "# atoms from \nODintegral"=→"Num Atoms - OD Integral" →"Last 40 numbers":dbl, "Chi-squared"=→"2D Fit Chi-squared":dbl)  [unwired: 2 in, 2 out]
                "2-D Fit Parameters" <- w176
                n75 = call "CalculateTemperature.vi"("Droptime (ms)"="?", "Isotope"="?", "2-D Fit Parameters"=w176) -> ("Avg. Temp"=→"?":ext)
              }
            }
          }
        }
        n76 = call "arrayaverage.vi"("Array int 32"=w37) -> ("Average"=→"Avg Atoms-Back":ext)
        n77 = Quotient & Remainder(x=w54, y="Save data every nth iteration") -> (x-y*floor(x/y)=w55:dbl)  [unwired: 1 out]
        "Strip chart counter" <- w55
        n78 = Equal?(x=w55, y=0) -> (x = y?=w52:bool)
        n79 = case shown="1" "Voltage\nMonitor\nControl" {
          tunnel: "Strip Chart\nerror in" -> [w87 w91 w99]
          tunnel: [w87 w90 w99] -> w58
          tunnel: "Monitor voltages?" -> [_ w89 _]
          tunnel: w52 -> [_ w88 _]
          frame 0, Default {
          }
          frame 1 {
            n80 = case shown="False" w89 {
              tunnel: w91 -> [w92 w97]
              tunnel: [w92 w96] -> w90
              tunnel: w88 -> [_ w93]
              frame False {
              }
              frame True {
                n81 = call "analog_input.vi"("save values?"=w93, "Voltage Log File Path"="Voltage Log File Path", 5:"Turn channels ON/OFF\n(works in real time)", "error in"=w97) -> ("error out"=w96:errorcluster, "Data display"=→"Analog Input \nVoltage Monitor":T1)  [unwired: 1 out]
              }
            }
          }
          frame 2 {
            # "Monitors Verdi temp\nand alerts user if\ntemp is too high."
            n82 = call "verditempalert.vi"() -> ()  [unwired: 1 in]
          }
        }
        "Strip Chart\nerror out" <- w58
        "iteration#" <- w54
      }
    }
    frame 2 {
      # "This frame stops the PixelFly camera, frees memory associated with the camera, and disowns the board."
      n83 = call <userlib>:"ShutDown.vi"() -> ("error out"=w228:errorcluster)  [unwired: 2 in, 1 out]
    }
  }
  "error out" <- w7
  "PixelFly Status" <- w1
  n84 = global write "check_pixelfly_status.vi" "PixelFly in Use?"(w1) -> ()
